vi "HEWH Channel Tester.vi"() -> ()   [LabVIEW 2019]
uses:
  Type Definitions/HEWH Sensor.ctl
  <vilib>/Analysis/NI_AALBase.lvlib
  <vilib>/Utility/file.llb/Write To Spreadsheet File (string).vi
  <vilib>/Utility/file.llb/Write To Spreadsheet File (DBL).vi
  Type Definitions/HEWH Equipment References.ctl
  Type Definitions/HEWH Tank Indicator.ctl
panel:
  out "Use Agilent?":bool
  out "Output Data":string[][](array[string])
  out "Calibration File Array":dbl[][](array[numeric])
  in  "Tab Control 2":T1(tab)
  in  "Panel 1":T2[][](array[typedef])=[[{"Mean"=0.0, " Std"=0.0, "Color Box"=8585007}, {"Mean"=0.0, " Std"=0.0, "Color Box"=8585007}, {"Mean"=0.0, " Std"=0.0, "Color Box"=8585007}, {"Mean"=0.0, " Std"=0.0, "Color Box"=8585007}, {"Mean"=0.0, " Std"=0.0, "Color Box"=8585007}, {"Mean"=0.0, " Std"=0.0, "Color Box"=8585007}], [{"Mean"=0.0, " Std"=0.0, "Color Box"=8585007}, {"Mean"=0.0, " Std"=0.0, "Color Box"=8585007}, {"Mean"=0.0, " Std"=0.0, "Color Box"=8585007}, {"Mean"=0.0, " Std"=0.0, "Color Box"=8585007}, {"Mean"=0.0, " Std"=0.0, "Color Box"=8585007}, {"Mean"=0.0, " Std"=0.0, "Color Box"=8585007}], [{"Mean"=0.0, " Std"=0.0, "Color Box"=8585007}, {"Mean"=0.0, " Std"=0.0, "Color Box"=8585007}, {"Mean"=0.0, " Std"=0.0, "Color Box"=8585007}, {"Mean"=0.0, " Std"=0.0, "Color Box"=8585007}, {"Mean"=0.0, " Std"=0.0, "Color Box"=8585007}, {"Mean"=0.0, " Std"=0.0, "Color Box"=8585007}]]
  in  "Panel 2":T2[][](array[typedef])=[[{"Mean"=0.0, " Std"=0.0, "Color Box"=8585007}, {"Mean"=0.0, " Std"=0.0, "Color Box"=8585007}, {"Mean"=0.0, " Std"=0.0, "Color Box"=8585007}, {"Mean"=0.0, " Std"=0.0, "Color Box"=8585007}, {"Mean"=0.0, " Std"=0.0, "Color Box"=8585007}, {"Mean"=0.0, " Std"=0.0, "Color Box"=8585007}], [{"Mean"=0.0, " Std"=0.0, "Color Box"=8585007}, {"Mean"=0.0, " Std"=0.0, "Color Box"=8585007}, {"Mean"=0.0, " Std"=0.0, "Color Box"=8585007}, {"Mean"=0.0, " Std"=0.0, "Color Box"=8585007}, {"Mean"=0.0, " Std"=0.0, "Color Box"=8585007}, {"Mean"=0.0, " Std"=0.0, "Color Box"=8585007}], [{"Mean"=0.0, " Std"=0.0, "Color Box"=8585007}, {"Mean"=0.0, " Std"=0.0, "Color Box"=8585007}, {"Mean"=0.0, " Std"=0.0, "Color Box"=8585007}, {"Mean"=0.0, " Std"=0.0, "Color Box"=8585007}, {"Mean"=0.0, " Std"=0.0, "Color Box"=8585007}, {"Mean"=0.0, " Std"=0.0, "Color Box"=8585007}]]
  in  "Panel 3":T2[][](array[typedef])=[[{"Mean"=0.0, " Std"=0.0, "Color Box"=8585007}, {"Mean"=0.0, " Std"=0.0, "Color Box"=8585007}, {"Mean"=0.0, " Std"=0.0, "Color Box"=8585007}, {"Mean"=0.0, " Std"=0.0, "Color Box"=8585007}, {"Mean"=0.0, " Std"=0.0, "Color Box"=8585007}, {"Mean"=0.0, " Std"=0.0, "Color Box"=8585007}], [{"Mean"=0.0, " Std"=0.0, "Color Box"=8585007}, {"Mean"=0.0, " Std"=0.0, "Color Box"=8585007}, {"Mean"=0.0, " Std"=0.0, "Color Box"=8585007}, {"Mean"=0.0, " Std"=0.0, "Color Box"=8585007}, {"Mean"=0.0, " Std"=0.0, "Color Box"=8585007}, {"Mean"=0.0, " Std"=0.0, "Color Box"=8585007}], [{"Mean"=0.0, " Std"=0.0, "Color Box"=8585007}, {"Mean"=0.0, " Std"=0.0, "Color Box"=8585007}, {"Mean"=0.0, " Std"=0.0, "Color Box"=8585007}, {"Mean"=0.0, " Std"=0.0, "Color Box"=8585007}, {"Mean"=0.0, " Std"=0.0, "Color Box"=8585007}, {"Mean"=0.0, " Std"=0.0, "Color Box"=8585007}]]
  in  "Num Samples":i32=5
  out "Data Sample":i32
  out "Power":T2={"Mean"=0.0, " Std"=0.0, "Color Box"=8585007}
  out "Tc Down":T2={"Mean"=0.0, " Std"=0.0, "Color Box"=8585007}
  out "Temperatures":T2[](array[typedef])=[{"Mean"=0.0, " Std"=0.0, "Color Box"=8585007}, {"Mean"=0.0, " Std"=0.0, "Color Box"=8585007}, {"Mean"=0.0, " Std"=0.0, "Color Box"=8585007}]
  out "Pressures":T2[](array[typedef])=[{"Mean"=0.0, " Std"=0.0, "Color Box"=8585007}, {"Mean"=0.0, " Std"=0.0, "Color Box"=8585007}, {"Mean"=0.0, " Std"=0.0, "Color Box"=8585007}]
  in  "Time Between Samples (Seconds)":u32
  in  "Tab Control":enum32{"DAQ Test", "Equipment"}(tab)
  in  "Test DAQ":bool
  in  "TC Max OK Val":dbl=400.0
  in  "PSI Min OK":dbl=100.0
  in  "TC Min OK Val":dbl=20.0
  in  "StDev Thresh":dbl=0.2
  in  "PSI Max OK":dbl=400.0
  in  "RTD Max OK":dbl=180.0
  in  "RTD Min OK":dbl=30.0
  in  "Calibration Path":path=path "C:/work/CalibrationFile.csv"
  in  "Equipment":T3={"MW100"="MW100", "AG34970"="A-34972A", "WT210"="WT210"}
  in  "OK":bool
  out "Calibration File?":bool
  in  "Calibration":T4(tab)
  in  "Select Panel to Calibrate":enum16{"Panel 1", "Panel 2", "Panel 3"}(ring)
  in  "Erase Cal File":bool
  in  "Calibrate":bool
  out "Temperature":dbl
  in  "Degrees F":dbl format="%^.3e"
  in  "Test Instrument":bool
  out "Calibration File Path":path
  out "Raw Data":dbl[][](array[numeric]) format="%_6g"
  out "Local Tank Display":T5 {"TC6" format="%.2g"; "TIN" format="%.2g"; "TOUT" format="%.2g"; "TC5" format="%.2g"; "TC4" format="%.2g"; "TC3" format="%.2g"; "TC2" format="%.2g"; "TC1" format="%.2g"}
  in  "error in (no error)":errorcluster
  # "This software is depricated"
  # "HEWH Pannel Channel Tester"
  # "DO NOT MODIFY WITHOUT PROPER PERMISSIONS"
  # "Instructions:\n1. Connect Fluke 525A or 525B (or equivalent) to the selected TC Panel\n2. Connect Fluke GPIB port to computer\n3. Erase old calibration file\n4. Select number of samples (300 default)\n4. Select the appropriate panel\n5. Set the instrument temperature (0,32,90 Degrees F)\n6. Press Calibrate TC's\n7. Repeat step 4 through 6"
  # "Step 1:"
  # "Step 2:"
  # "Step 3:"
  # "Step 5:"
  # "Step 6:"
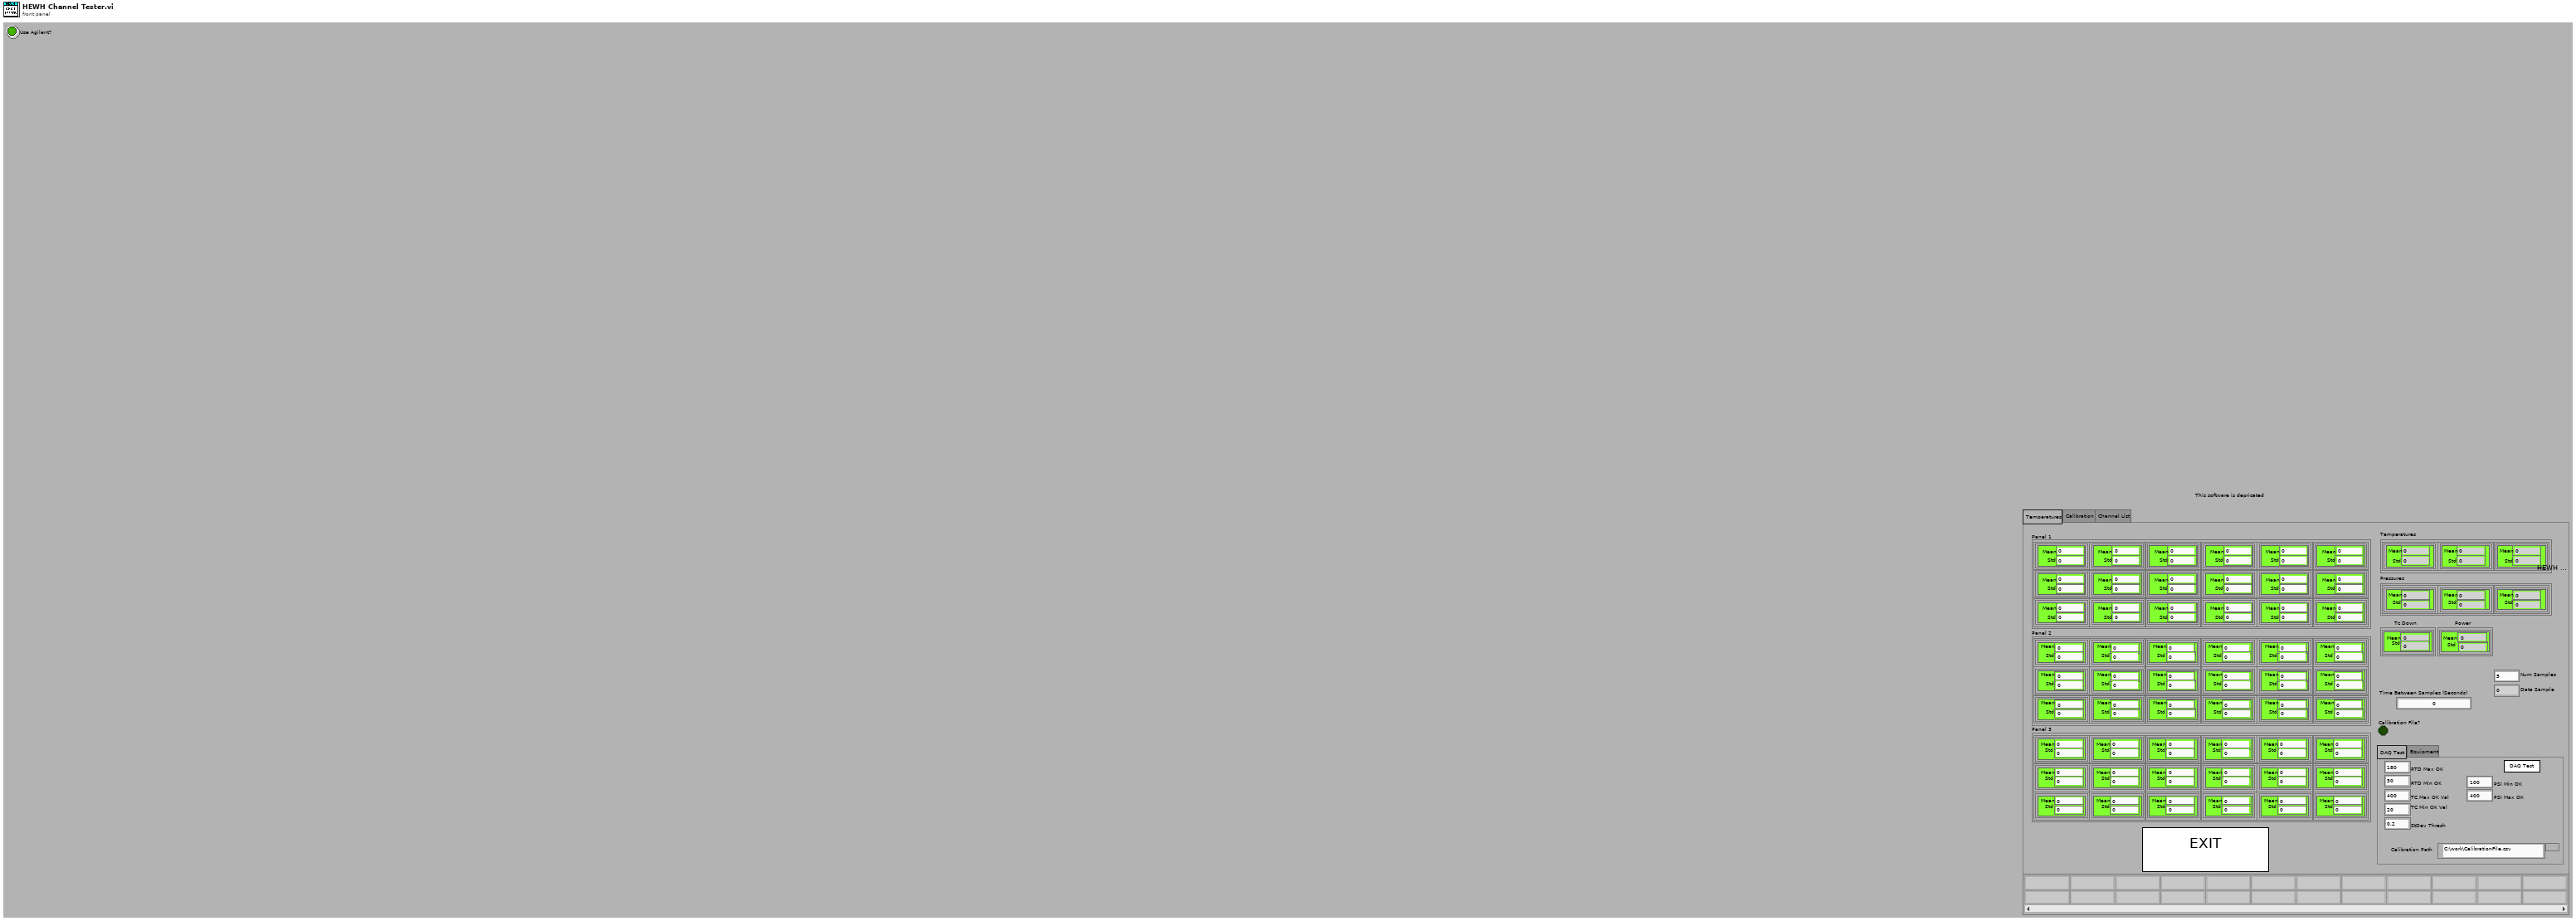
[diagram p1: front panel]
types:
  T1 = enum32{"Temperatures", "Calibration", "Channel List"}
  T2 = typedef "HEWH Sensor.ctl" = cluster{"Mean":dbl, " Std":dbl, "Color Box":u32}
  T3 = typedef "HEWH Equipment References.ctl" = cluster{"MW100":refnum<visa-resource-name>, "AG34970":refnum<visa-resource-name>, "WT210":refnum<visa-resource-name>}
  T4 = enum32{"Calibration Sequence", "Write File", "Debug"}
  T5 = typedef "HEWH Tank Indicator.ctl" = cluster{"TC1":dbl, "TC2":dbl, "TC3":dbl, "TC4":dbl, "TC5":dbl, "TIN":dbl, "TOUT":dbl, "TC6":dbl, "TC6-Color":u32, "TC5-Color":u32, "TC4-Color":u32, "TC3-Color":u32, "TC2-Color":u32, "TC1-Color":u32, "RTD-Out":u32, "RTD-In":u32}
  T6 = enum32{"invalid app kind", "Development System", "Run Time System", "Student Edition", "Embedded LabVIEW", "Evaluation", "Custom"}
  T7 = enum32{"Invalid", "Standard", "Closed", "Hidden", "Minimized", "Maximized"}
  T8 = cluster{"Core":cluster{"Current VI Reference":refnum<vi>, "Close Panel on Exit?":bool}, "Num Samples":i32, "HEWH Power":bool, "Test Data Array":T2[], "Channel List":string}
  T9 = cluster{"Current VI Reference":refnum<vi>, "Close Panel on Exit?":bool}
  T10 = typedef "HEWH Agilent Cluster.ctl" = cluster{"Label":string, "Agilent Channel":string, "Panel ID":string, "Source":string, "Temperature":dbl}
  T11 = typedef "FileVersionInformation.ctl" = cluster{"FileVersion":string, "ProductName":string, "InternalName":string, "CompanyName":string, "LegalCopyright":string, "FileDescription":string}
  T12 = typedef "HEWH Output Information.ctl" = cluster{"TR Number:":string, "Lab ID:":string, "Calibration Array":string[][], "Test Number:":string, "Model:":string, "Serial Number:":string, "Build:":string, "Ambient Temp SetPoint:":string, "Test Station:":string, "Frequency:":string, "Ambient RH:":string, "Comments:":string, "Technician:":string, "Engineer:":string, "Date:":string, "Version:":string, "Computer:":string, "Filename":string, "Heating Mode":string, "FileVersionInfo":T11, "File Initialization Array":string[][], "File Path":path, "Computer IP Address:":string, "Agilent Channel List":string, "Agilent Cluster Array":T13[], "Calibration Coefficients":dbl[][], "Agilent Raw Cluster Array":T13[], "Data Table":string[][], "RLT Station?":bool, "Scan Rate Adjust":dbl, "Start Gallons":dbl, "Last GPM Reading":dbl, "PowerData":T14, "Draw Count":i32, "Draw Patten Setup":T15, "Draw Until Condition":T17, "TC Tree":dbl[], "Starting Temp Decline Temp":dbl, "Full Data Table":string[][], "Max RTD Temp\nDuring Draw":dbl, "Min RTD Temp\nDuring Draw":dbl, "RTD Max Min Array":dbl[][], "Draw Start Time":dbl, "Draw Statistics":dbl[][], "Last Temp Reading":dbl, "Custom Test Array":T18[], "Delay Start Time":dbl, "Condition Cluster Output":T20, "Valve % Open":dbl, "PreDraw Data Table":string[][]}
  T13 = typedef "Agilent Cluster.ctl" = cluster{"Label":string, "Agilent Channel":string, "Panel ID":string, "Source":string, "Temperature":dbl}
  T14 = typedef "PowerData.ctl" = cluster{"Voltage (Volts)":dbl, "Current (Amps)":dbl, "Power (Watts)":dbl, "WattHours (Wh)":dbl, "TC Tree (AVG)":dbl, "Flow Rate (GPM)":dbl, "Gallons (Gal)":dbl, "RTD Out (Deg F)":dbl, "TC Down":dbl}
  T15 = typedef "Draw Pattern Setup.ctl" = cluster{"Dispense Times":dbl[], "Total Gallons Schedule":dbl[], "Flow Rate Schedule ":dbl[], "Incoming Water Temperature":dbl[], "PreDraw Pattern":dbl[][], "Repeat":bool, "24 Hour PreDraw":T16, "Draw Until?":bool[]}
  T16 = typedef "PreDraw.ctl" = enum16{"Zero Pre-Draws", "One Pre- Draws", "Two Pre-Draws", "Three Pre-Draws", ""}
  T17 = typedef "PowerElements.ctl" = cluster{"UE":bool, "LE":bool, "COMP":bool, "FANS":bool}
  T18 = typedef "Custom Test.ctl" = cluster{"Custom Test Value":dbl, "Flow Rate (GPM)":dbl, "Incoming Water  Temperature ":dbl, "Action Type":T19}
  T19 = typedef "Custom Test - Conditions.ctl" = enum16{"", "Set Set Point", "Set to Heat Pump", "Set to Hybrid", "Set to High Demand", "Set to Electric", "Set to Vacation", "Set to Northern Climate", "Check Mode", "Start Test Timer", "Test Timer < Value", "Test Timer > Value", "Check - Test Timer", "Check - Cutout", "Check - Comp ON", "Check - Comp OFF", "Check - Comp & Fan ON", "Check - Comp & Fan OFF", "Check - LE ON", "Check - LE OFF", "Check - UE ON", "Check - UE OFF", "Check - Elapsed Time (sec)", "Check - Mean Tank Temp", "Check - RTD Out Temp Reduction", "Check - RTD Out Temp", "Draw - Elapsed Time (sec)", "Draw - Gallon Target", "Draw - Until Comp", "Draw - Until Comp & Fan", "Draw - Until LE", "Draw - Until UE", "Draw - Any Heat Source", "Draw - Until RTD Out Temp", "Draw - Until RTD Out Temp Reduction", "Draw - Until Mean Tank Temp", "Wait - Cutout", "Wait - Comp ON", "Wait - Comp & Fan ON", "Wait - Comp OFF", "Wait - Comp & Fan OFF", "Wait - LE ON", "Wait - LE OFF", "Wait - UE ON", "Wait - UE OFF", "Wait - Elapsed Time (sec)", "Wait - RTD Out Temp", "Wait - RTD Out Temp Reduction", "Wait - Mean Tank Temp", "Terminate - Comp ON", "Terminate - Comp & Fan ON", "Terminate - Comp OFF", "Terminate - Comp & Fan OFF", "Terminate - LE ON", "Terminate - LE OFF", "Terminate - UE ON", "Terminate - UE OFF", "Terminate - RTD Out Temp", "Terminate - Mean Tank Temp", "Terminate - UE or LE ON", "Terminate - UE or LE OFF", "Terminate - Cutout", "Repeat"}
  T20 = typedef "Termination Condition Cluster.ctl" = cluster{"Decrease RTD Output\nTemperature Bool":bool, "RTD Out Temperature Bool":bool, "Use Time Bool":bool, "RTD Out Temperature":T21, "Decrease Outlet Temperature By (RTD Out)":T21, "Time (Seconds)":T21, "Draw Until Condition":T17, "Start Draw Until Specific Bool":bool, "Return Output Bool":bool, "Draw Until Any Heat Bool":bool, "Mean Tank Temperature Bool":bool, "Mean Tank Temperature":T21, "Comp OFF":bool, "Comp & Fan OFF":bool, "UE OFF":bool, "LE OFF":bool}
  T21 = typedef "DBL.ctl" = dbl
  T22 = typedef "EquipReferences.ctl" = cluster{"MW100":refnum<visa-resource-name>, "AG34970":refnum<visa-resource-name>, "WT210":refnum<visa-resource-name>}
  T23 = typedef "User Controls.ctl" = cluster{"Main Power Control":bool, "Out VLV":enum8{"CLOSE", "OPEN"}, "Expansion Tank?":bool, "In VLV":enum8{"OPEN", "CLOSE"}, "Drain VLV":enum8{"OPEN", "CLOSE"}, "Flow Totalizer Control":bool, "Intellifaucet Temperature":dbl, "Percent Flow":dbl, "Safe Mode":bool, "In VLV B":enum8{"OPEN", "CLOSE"}, "Drain VLV B":enum8{"OPEN", "CLOSE"}, "Out VLV B":enum8{"CLOSE", "OPEN"}, "In VLV C":enum8{"OPEN", "CLOSE"}, "Drain VLV C":enum8{"OPEN", "CLOSE"}, "Out VLV C":enum8{"CLOSE", "OPEN"}, "In VLV D":enum8{"OPEN", "CLOSE"}, "Drain VLV D":enum8{"OPEN", "CLOSE"}, "Out VLV D":enum8{"CLOSE", "OPEN"}, "GEA2?":bool, "Use Agilent?":bool, "Valve Set A":enum16{"Heating", "Purge", "Resting", "Draw"}, "Valve Set B":enum16{"Heating", "Purge", "Resting", "Draw"}, "Valve Set C":enum16{"Heating", "Purge", "Resting", "Draw"}, "Valve Set D":enum16{"Heating", "Purge", "Resting", "Draw"}}
  T24 = typedef "PowerAnalyzer.ctl" = enum16{"OSI", "WT210"}
  T25 = cluster{"Core":cluster{"Current VI Reference":refnum<vi>, "Close Panel on Exit?":bool}, "FileVersionInfo Out 2":T11, "Data File Directory":path, "FileInit Cluster":T12, "Equipment VISA":T22, "User Controls":T23, "POWER":T17, "Save Data":string[][], "Calibration File":path, "Power Analyzer":T24}
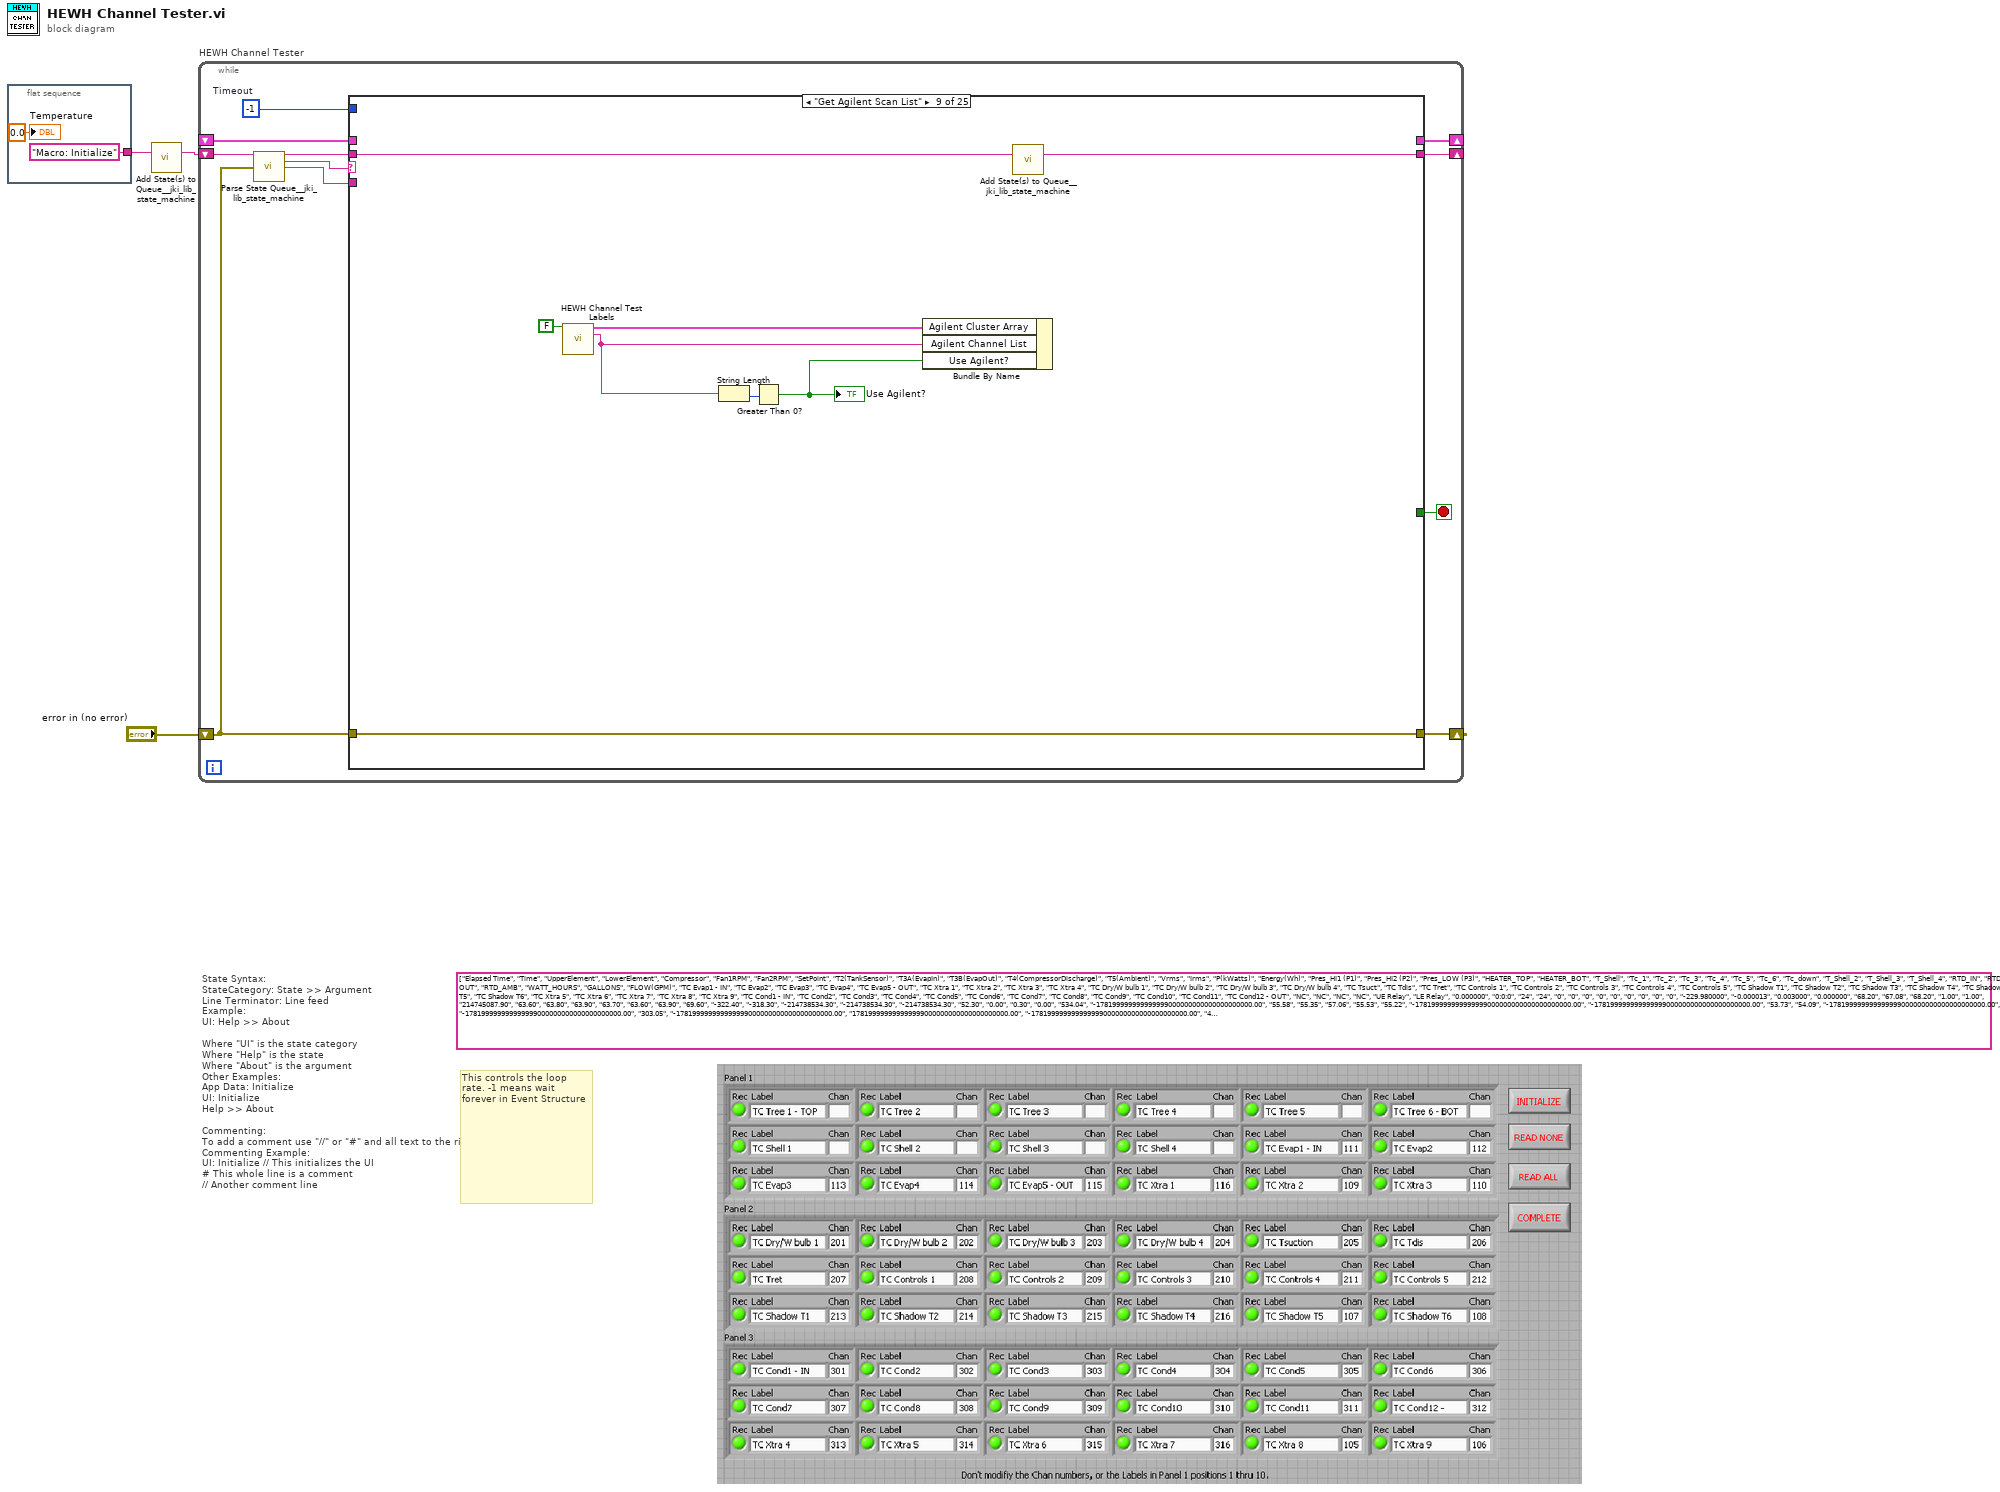
[diagram p0: block diagram]
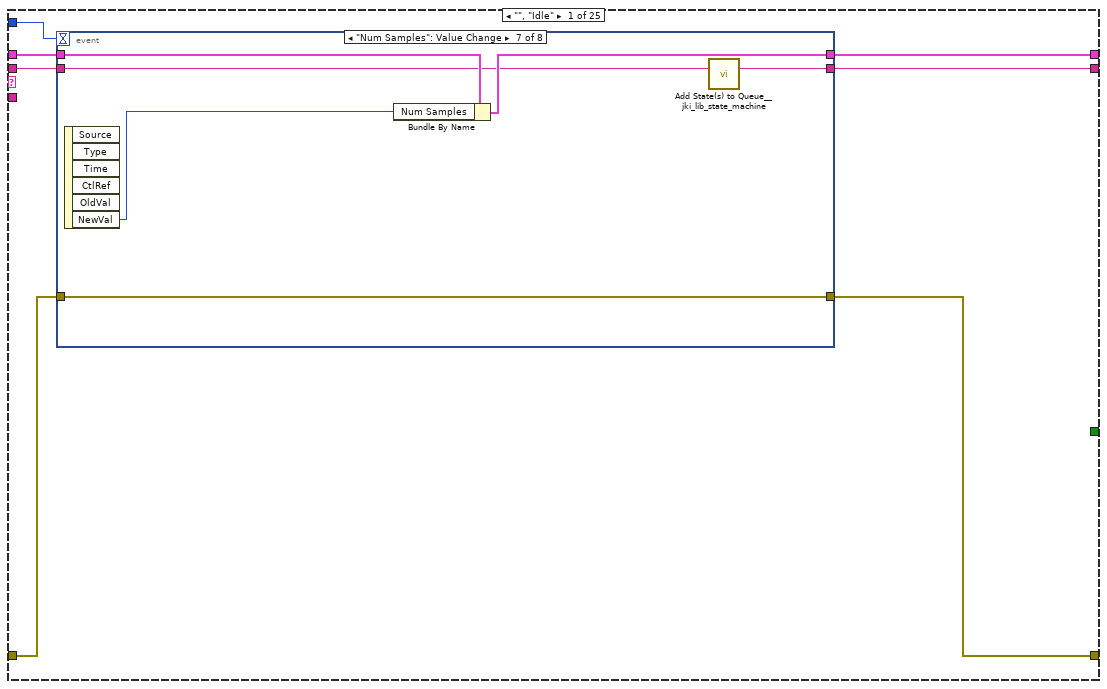
[diagram p2: hidden frame]
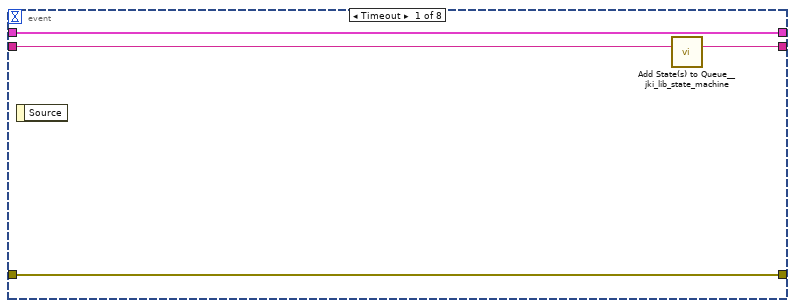
[diagram p3: hidden frame]
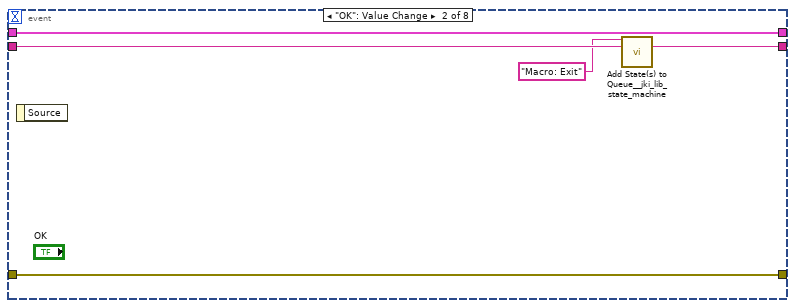
[diagram p4: hidden frame]
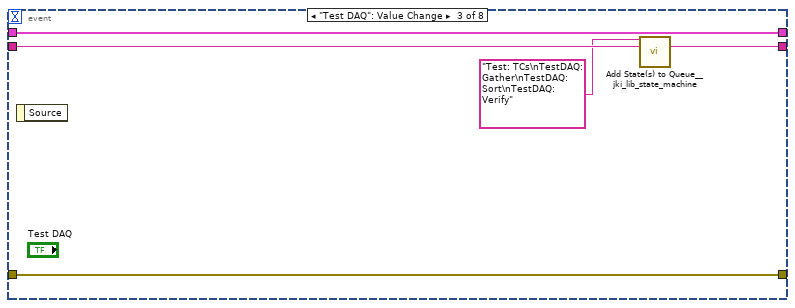
[diagram p5: hidden frame]
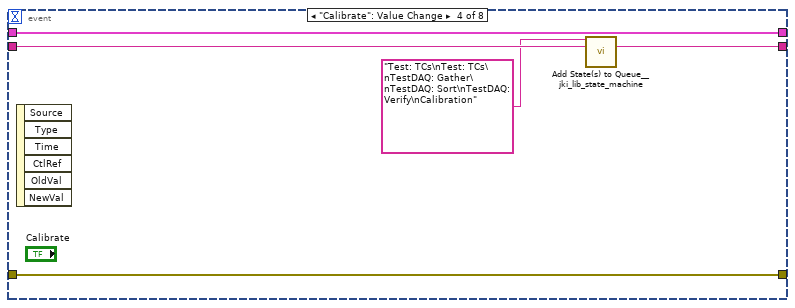
[diagram p6: hidden frame]
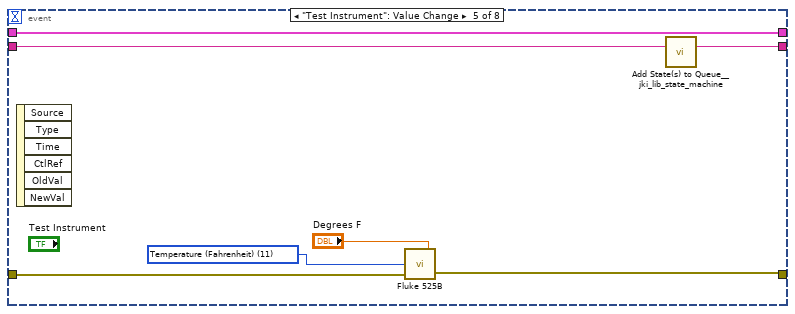
[diagram p7: hidden frame]
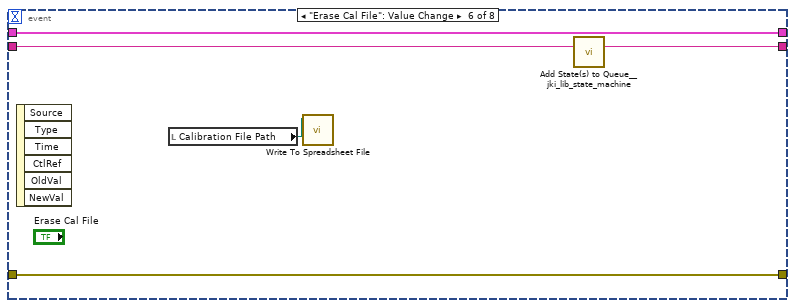
[diagram p8: hidden frame]
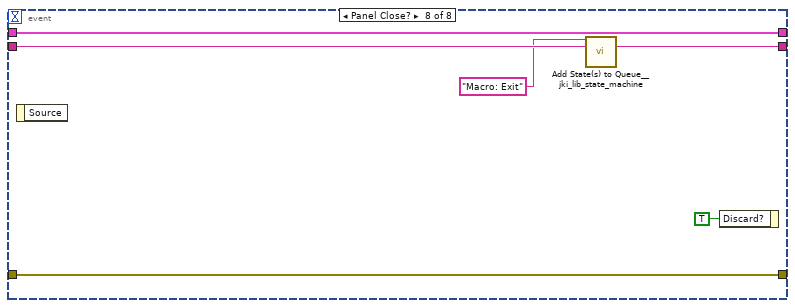
[diagram p9: hidden frame]
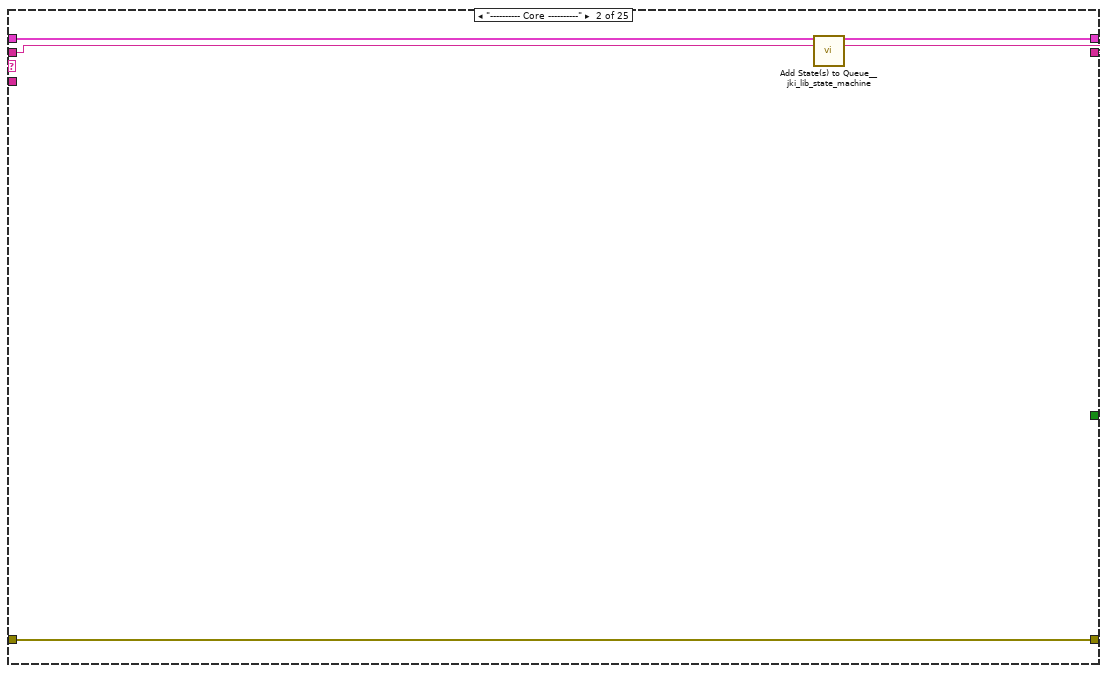
[diagram p10: hidden frame]
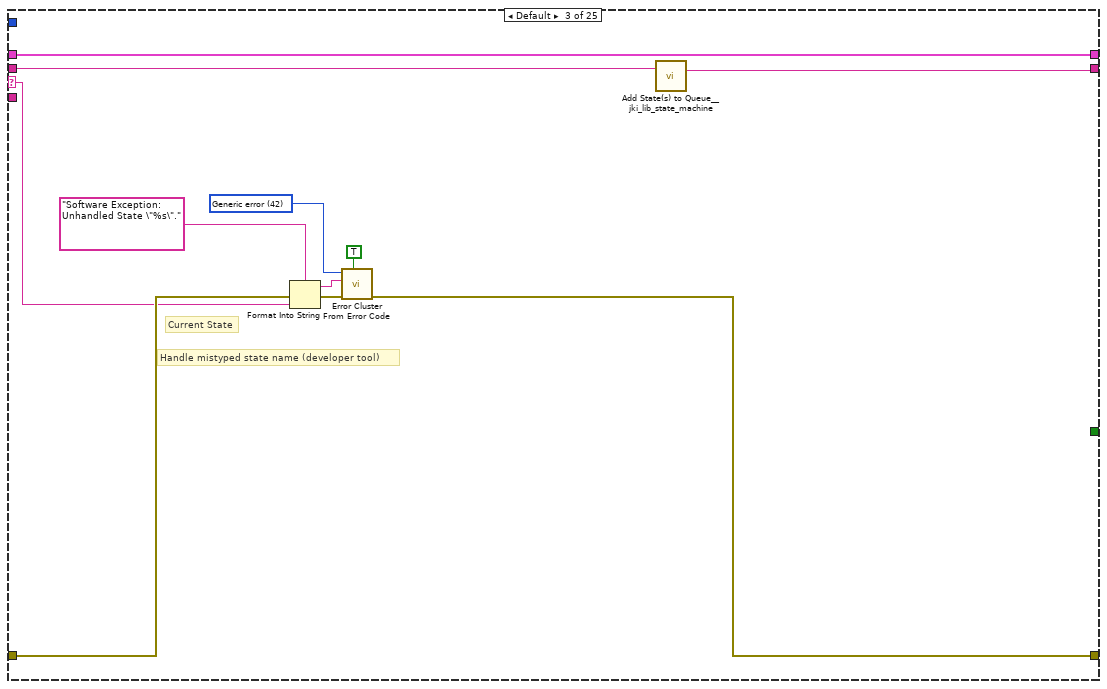
[diagram p11: hidden frame]
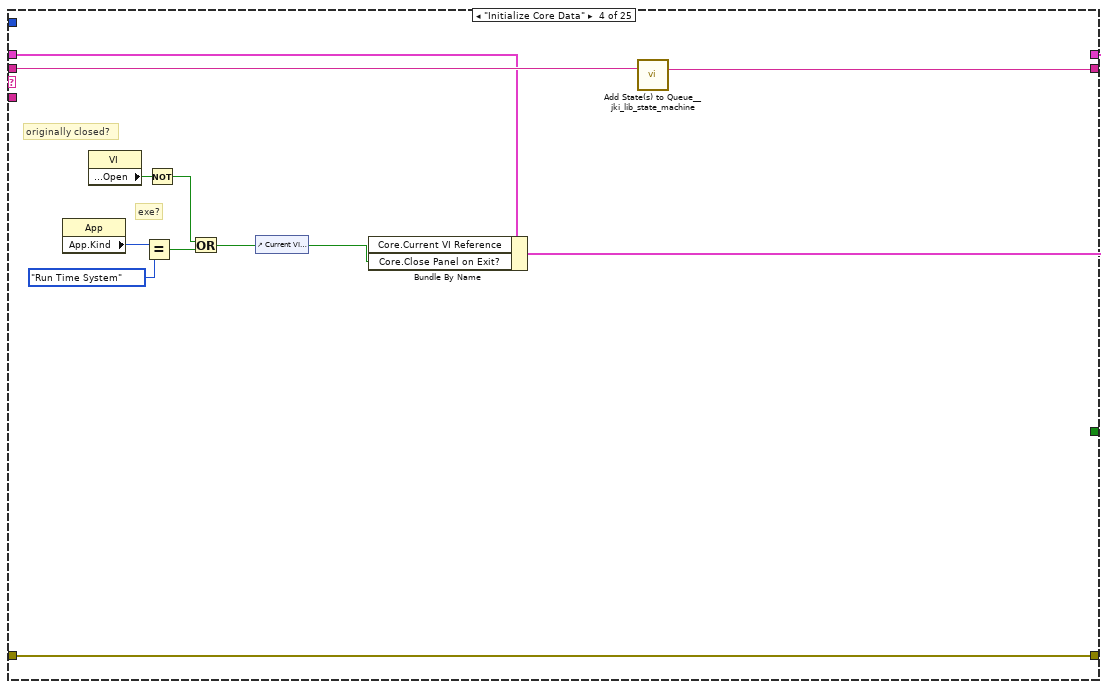
[diagram p12: hidden frame]
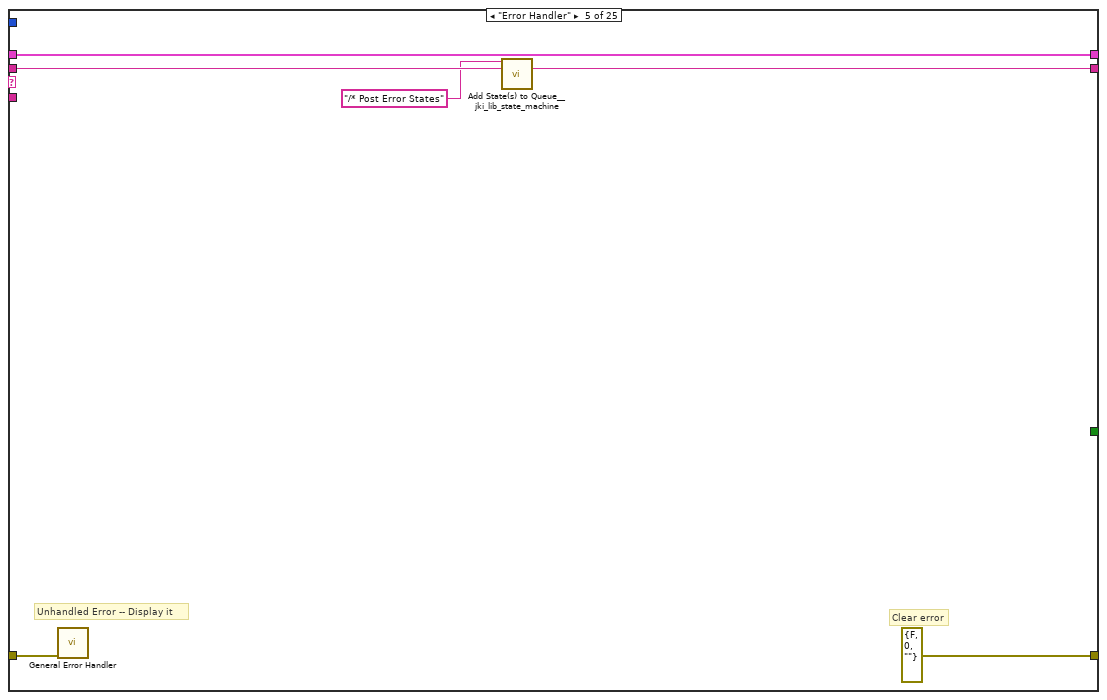
[diagram p13: hidden frame]
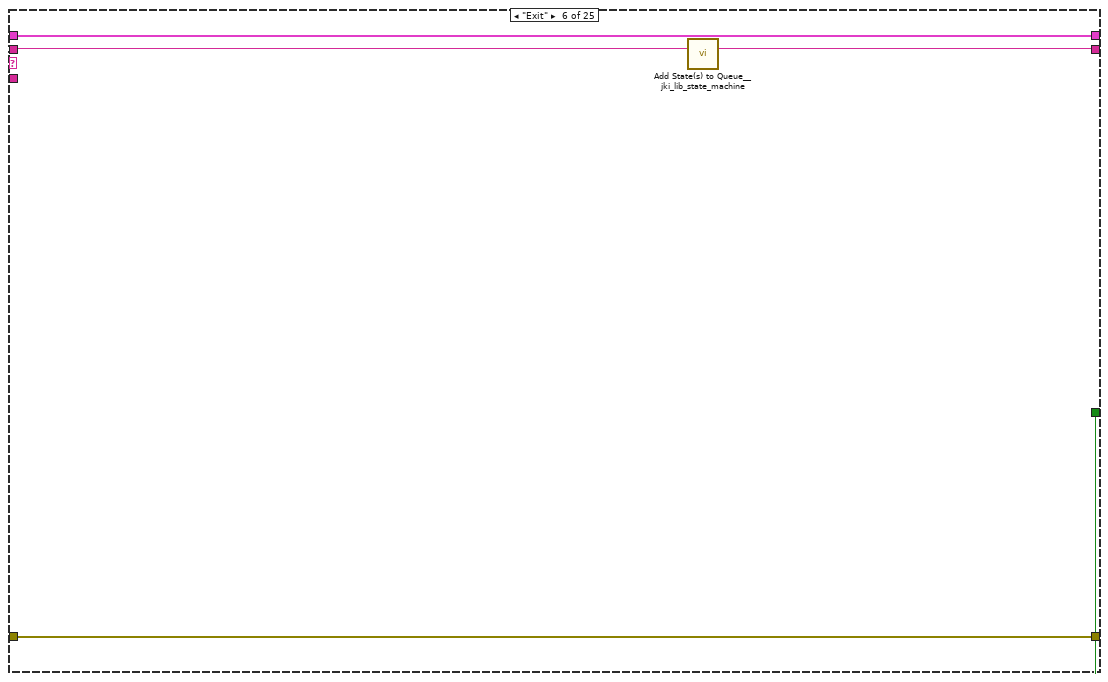
[diagram p14: hidden frame]
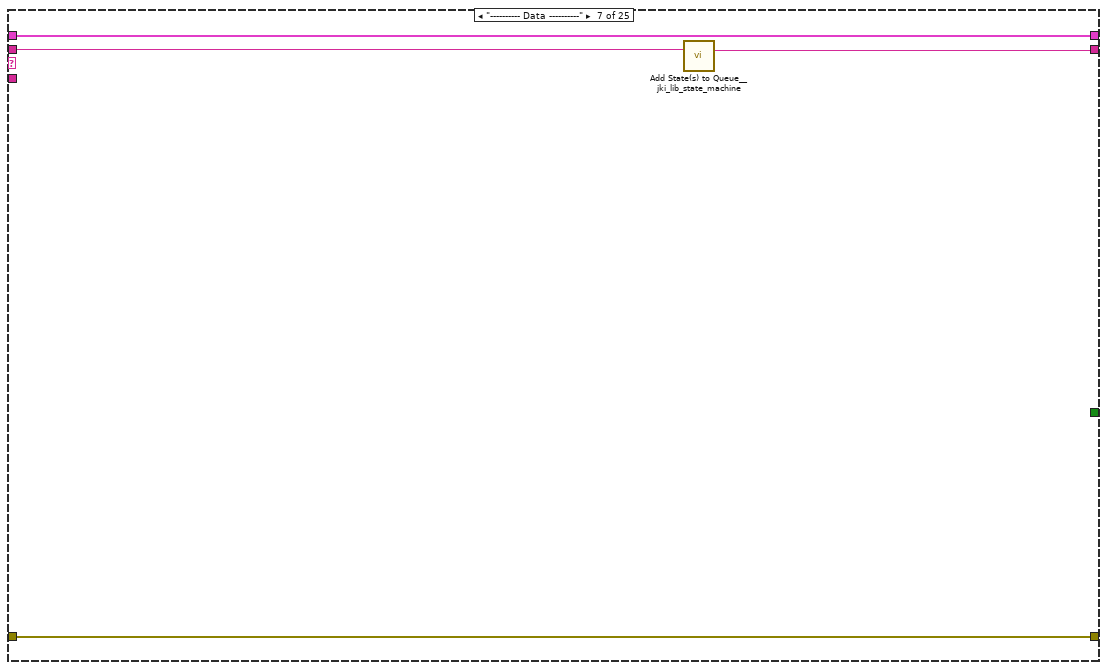
[diagram p15: hidden frame]
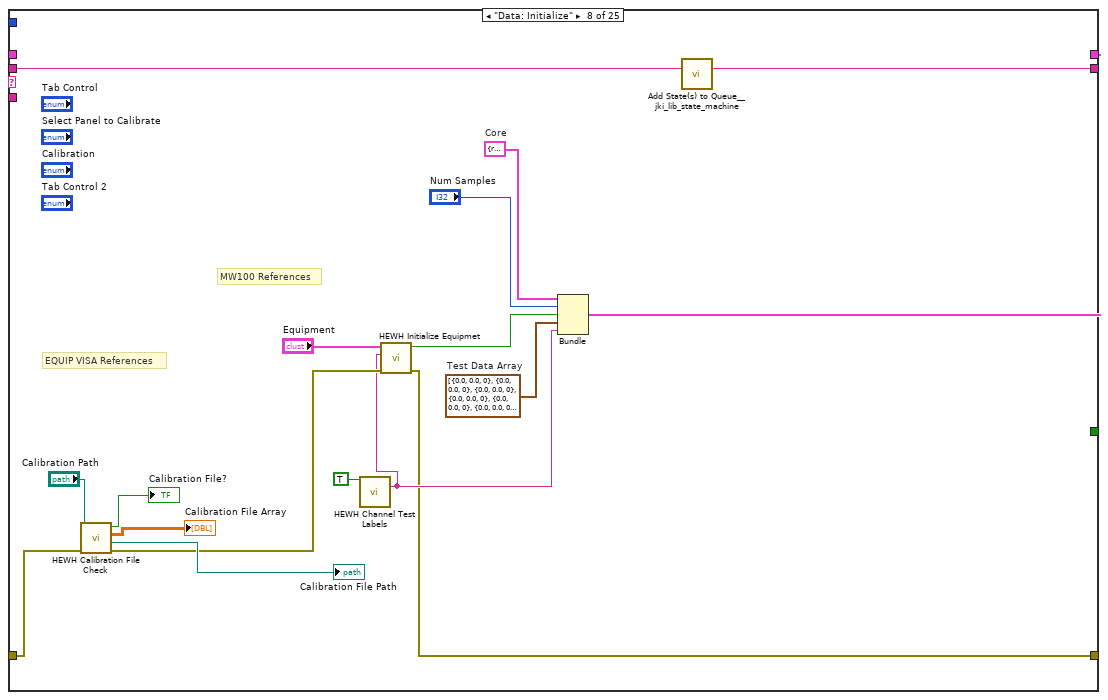
[diagram p16: hidden frame]
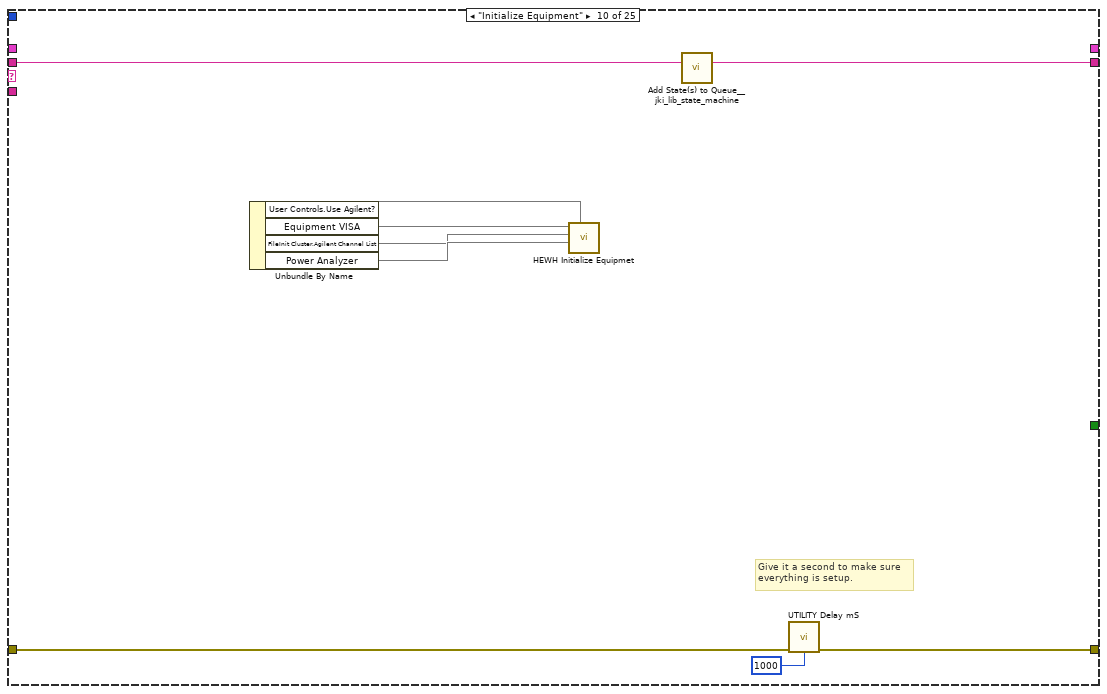
[diagram p17: hidden frame]
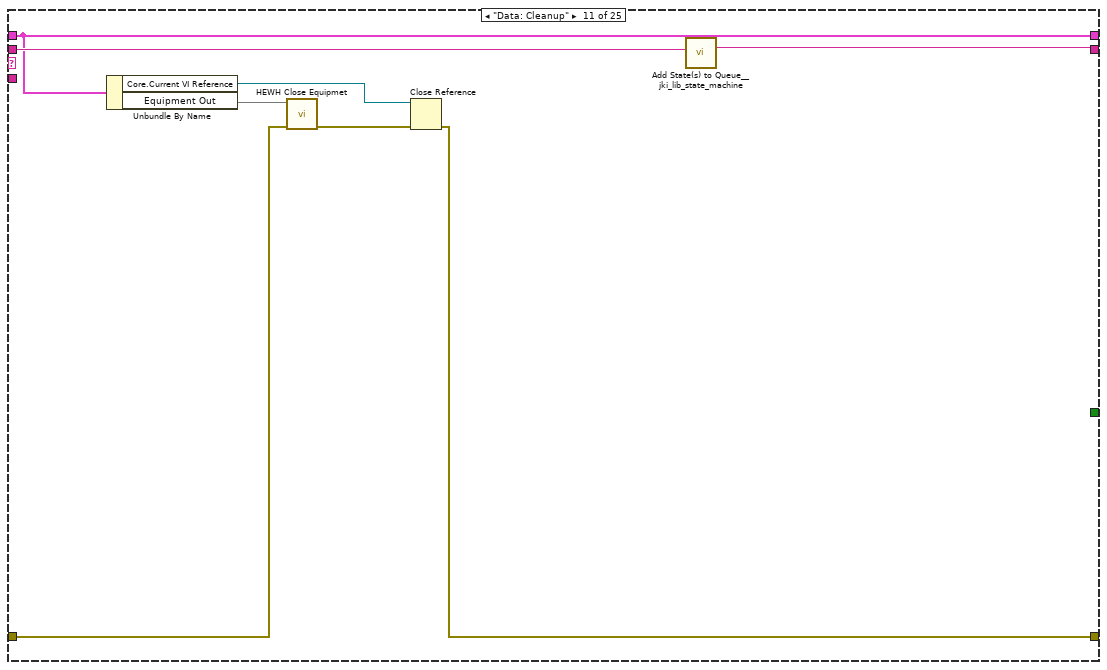
[diagram p18: hidden frame]
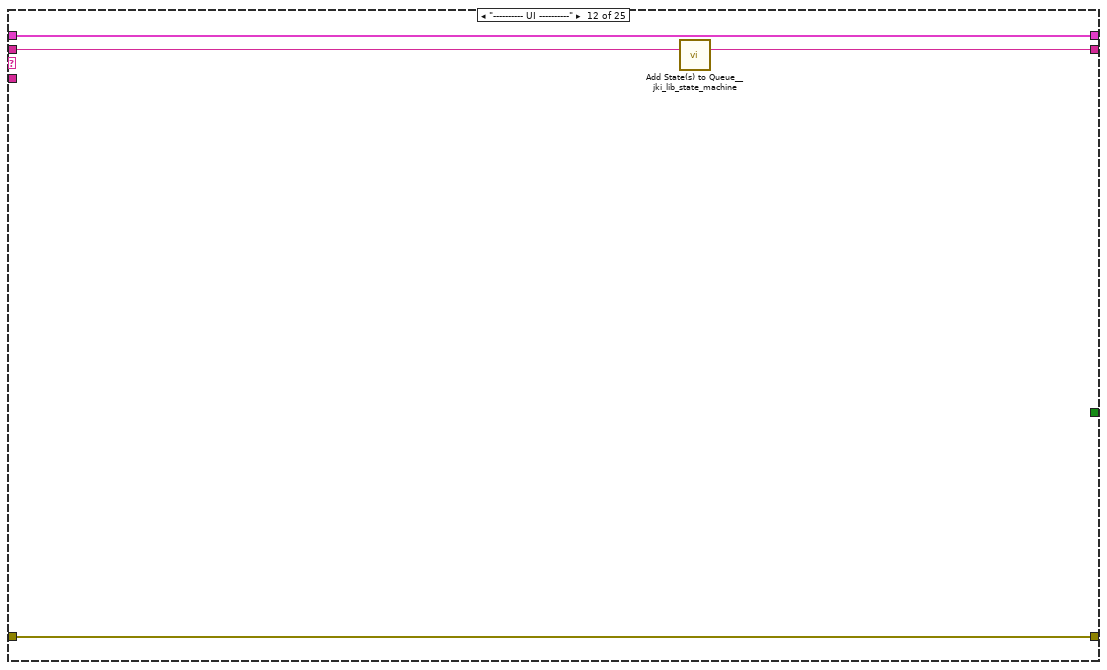
[diagram p19: hidden frame]
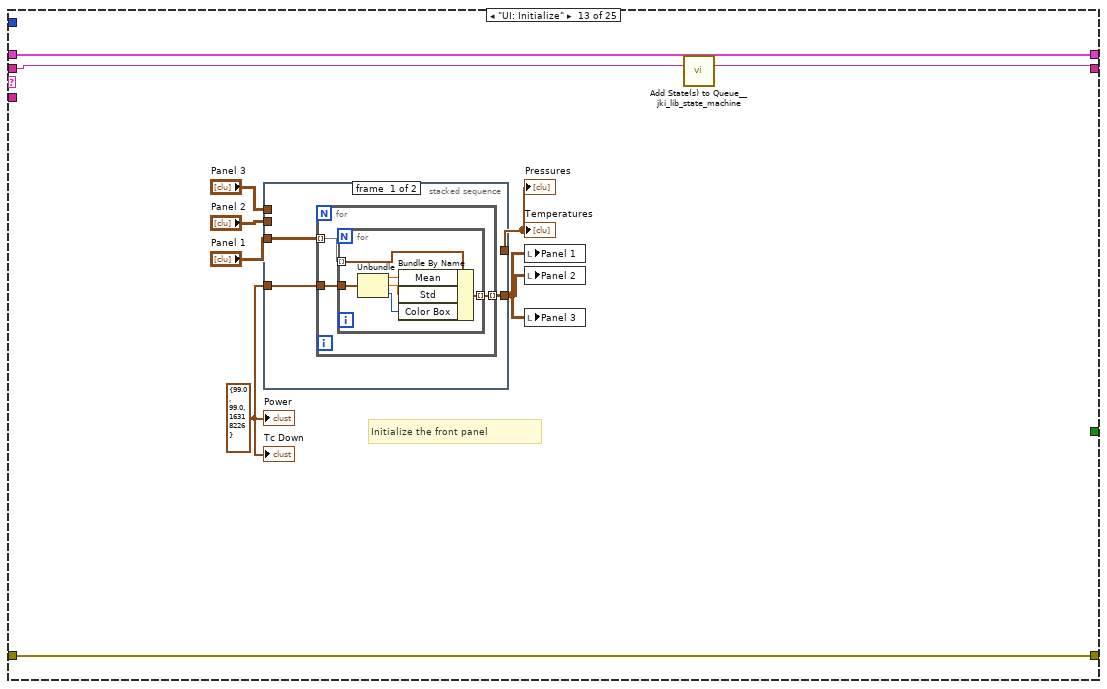
[diagram p20: hidden frame]
diagram:
  (unwired) string[][] [["Elapsed Time", "Time", "UpperElement", "LowerElement", "Compressor", "Fan1RPM", "Fan2RPM", "SetPoint", "T2(TankSensor)", "T3A(EvapIn)", "T3B(EvapOut)", "T4(CompressorDischarge)", "T5(Ambient)", "Vrms", "Irms", "P(kWatts)", "Energy(Wh)", "Pres_HI1 (P1)", "Pres_HI2 (P2)", "Pres_LOW (P3)", "HEATER_TOP", "HEATER_BOT", "T_Shell", "Tc_1", "Tc_2", "Tc_3", "Tc_4", "Tc_5", "Tc_6", "Tc_down", "T_Shell_2", "T_Shell_3", "T_Shell_4", "RTD_IN", "RTD_OUT", "RTD_AMB", "WATT_HOURS", "GALLONS", "FLOW(GPM)", "TC Evap1 - IN", "TC Evap2", "TC Evap3", "TC Evap4", "TC Evap5 - OUT", "TC Xtra 1", "TC Xtra 2", "TC Xtra 3", "TC Xtra 4", "TC Dry/W bulb 1", "TC Dry/W bulb 2", "TC Dry/W bulb 3", "TC Dry/W bulb 4", "TC Tsuct", "TC Tdis", "TC Tret", "TC Controls 1", "TC Controls 2", "TC Controls 3", "TC Controls 4", "TC Controls 5", "TC Shadow T1", "TC Shadow T2", "TC Shadow T3", "TC Shadow T4", "TC Shadow T5", "TC Shadow T6", "TC Xtra 5", "TC Xtra 6", "TC Xtra 7", "TC Xtra 8", "TC Xtra 9", "TC Cond1 - IN", "TC Cond2", "TC Cond3", "TC Cond4", "TC Cond5", "TC Cond6", "TC Cond7", "TC Cond8", "TC Cond9", "TC Cond10", "TC Cond11", "TC Cond12 - OUT", "NC", "NC", "NC", "NC", "UE Relay", "LE Relay"], ["0.000000", "0:0:0", "24", "24", "0", "0", "0", "0", "0", "0", "0", "0", "0", "-229.980000", "-0.000013", "0.003000", "0.000000", "68.20", "67.08", "68.20", "1.00", "1.00", "214745087.90", "63.60", "63.80", "63.90", "63.70", "63.60", "63.90", "69.60", "-322.40", "-318.30", "-214738534.30", "-214738534.30", "-214738534.30", "52.30", "0.00", "0.30", "0.00", "534.04", "-178199999999999999000000000000000000000.00", "55.58", "55.35", "57.06", "55.53", "55.22", "-178199999999999999000000000000000000000.00", "-178199999999999999000000000000000000000.00", "53.73", "54.09", "-178199999999999999000000000000000000000.00", "-178199999999999999000000000000000000000.00", "303.05", "-178199999999999999000000000000000000000.00", "178199999999999999000000000000000000000.00", "-178199999999999999000000000000000000000.00", "460.73", "626.99", "-178199999999999999000000000000000000000.00", "178199999999999999000000000000000000000.00", "-178199999999999999000000000000000000000.00", "131.37", "178199999999999999000000000000000000000.00", "-178199999999999999000000000000000000000.00", "-178199999999999999000000000000000000000.00", "409.13", "259.86", "-178199999999999999000000000000000000000.00", "178199999999999999000000000000000000000.00", "-178199999999999999000000000000000000000.00", "-57.06", "62.09", "61.89", "61.87", "62.14", "62.63", "178199999999999999000000000000000000000.00", "-178199999999999999000000000000000000000.00", "178199999999999999000000000000000000000.00", "-70.58", "-178199999999999999000000000000000000000.00", "178199999999999999000000000000000000000.00", "-178199999999999999000000000000000000000.00", "393.52", "116.86", "83.34", "59.96", "0", "0"]] ("Output Data")
  # "State Syntax:\nStateCategory: State >> Argument\nLine Terminator: Line feed\nExample:\nUI: Help >> About\n\nWhere \"UI\" is the state category\nWhere \"Help\" is the state\nWhere \"About\" is the argument\nOther Examples:\nApp Data: Initialize\nUI: Initialize\nHelp >> About\n\nCommenting:\nTo add a comment use \"//\" or \"#\" and all text to the right will be ignored\nCommenting Example:\nUI: Initialize // This initializes the UI\n# This whole line is a comment\n// Another comment line"
  # "This controls the loop rate. -1 means wait forever in Event Structure"
  n1 = flat-sequence {
    tunnel: ["Macro: Initialize"] -> w1
    frame #0 {
      "Temperature" <- 0.0 ("Temp Counter")
    }
  }
  n2 = call <vilib>:"Add State(s) to Queue__jki_lib_state_machine.vi"("State(s) in (\"\")"=w1) -> ("States Out"=w3:string)  [unwired: 14 in]
  n3 = while "HEWH Channel Tester" {
    shift-right: [w9] -> _
    shift-left: _ -> [w8]
    shift-right: [w12] -> _
    shift-left: "error in (no error)" -> [w6]
    shift-right: [w11] -> _
    shift-left: w3 -> [w13]
    stop <- w10 stop-if-true
    w7 = -1  # Timeout
    # "Template Copyright © 2008 JKI - http://jkisoft.com/state-machine"
    n4 = call <vilib>:"Parse State Queue__jki_lib_state_machine.vi"("State Queue"=w13, "Error In (no error)"=w6) -> ("Remaining States"=w15:string, "Current State"=w16:string, "Arguments"=w14:string)  [unwired: 11 in]
    n5 = case shown="\"Get Agilent Scan List\"" w16 {
      selector: w16 -> [_ _ w73 _ _ _ _ _ _ _ _ _ _ _ _ _ _ _ _ _ _ _ _ _ _]
      tunnel: w15 -> [w23 w70 w71 w93 w99 w104 w108 w125 w133 w143 w151 w155 w165 w188 w199 w225 w230 w240 w244 w248 w252 w263 w289 w374 w412]
      tunnel: w14 -> [_ _ _ _ _ _ _ _ _ _ _ _ _ w183 w193 _ _ _ _ _ _ _ _ _ _]
      tunnel: w8 -> [w21 w67 w75 w84 w96 w102 w105 _ _ _ w147 w152 w163 w186 w195 w222 w227 w237 w241 w245 w249 w259 w286 w371 w410]
      tunnel: [w20 w68 w77 w90 errorcluster {"status"=FALSE, "code"=0, "source"=""} ("error out") w101 w106 w110 w131 w134 w148 w153 w162 w184 w196 w223 w228 w238 w242 w246 w250 w261 w287 w372 w406] -> w12
      tunnel: w6 -> [w19 w68 w76 w90 w95 w101 w106 w114 w131 w135 w144 w153 w162 w185 w197 w223 w228 w238 w242 w246 w250 w255 w287 w372 w407]
      tunnel: [w22 w69 w72 w92 w98 w103 w107 w124 w132 w142 w150 w154 w164 w187 w198 w224 w229 w239 w243 w247 w251 w262 w288 w373 w411] -> w11
      tunnel: [_ _ _ _ _ TRUE _ _ _ _ _ _ _ _ _ _ _ _ _ _ _ _ _ _ _] -> w10
      tunnel: [w18 w67 w75 w91 w96 w102 w105 w123 _ _ w147 w152 w163 w186 w195 w222 w227 w237 w241 w245 w249 w257 w286 w371 w410] -> w9
      tunnel: w7 -> [w17 _ _ _ _ _ _ _ _ _ _ _ _ _ _ _ _ _ _ _ _ _ _ _ _]
      frame "", "Idle" {
        n6 = event shown="[6] \"Num Samples\": Value Change" {
          selector: _ -> [_ _ _ _ _ _ _ _]
          dyn-events: _ -> [_ _ _ _ _ _ _ _]
          timeout: w17 -> [_ _ _ _ _ _ _ _]
          tunnel: w23 -> [w27 w32 w37 w42 w48 w53 w58 w66]
          tunnel: [w26 w31 w36 w41 w49 w52 w57 w65] -> w22
          tunnel: w21 -> [w24 w29 w34 w39 w47 w54 w60 w63]
          tunnel: [w25 w30 w35 w40 w43 w51 w56 w64] -> w20
          tunnel: w19 -> [w25 w30 w35 w40 w44 w51 w56 w64]
          tunnel: [w24 w29 w34 w39 w47 w54 w59 w63] -> w18
          event Timeout {
            n7 = event-data() -> ()  [unwired: 1 in, 1 out]
            n8 = call <vilib>:"Add State(s) to Queue__jki_lib_state_machine.vi"("State(s) in (\"\")"=w27) -> ("States Out"=w26:string)  [unwired: 14 in]
          }
          event "OK": Value Change {
            n9 = event-data() -> ()  [unwired: 1 in, 1 out]
            n10 = call <vilib>:"Add State(s) to Queue__jki_lib_state_machine.vi"("State(s) in Front (\"\")"="Macro: Exit", "State(s) in (\"\")"=w32) -> ("States Out"=w31:string)  [unwired: 13 in]
          }
          event "Test DAQ": Value Change {
            n11 = event-data() -> ()  [unwired: 1 in, 1 out]
            n12 = call <vilib>:"Add State(s) to Queue__jki_lib_state_machine.vi"("State(s) in Front (\"\")"="Test: TCs\nTestDAQ: Gather\nTestDAQ: Sort\nTestDAQ: Verify", "State(s) in (\"\")"=w37) -> ("States Out"=w36:string)  [unwired: 13 in]
          }
          event "Calibrate": Value Change {
            n13 = event-data() -> ()  [unwired: 1 in, 6 out]
            n14 = call <vilib>:"Add State(s) to Queue__jki_lib_state_machine.vi"("State(s) in Front (\"\")"="Test: TCs\nTest: TCs\nTestDAQ: Gather\nTestDAQ: Sort\nTestDAQ: Verify\nCalibration", "State(s) in (\"\")"=w42) -> ("States Out"=w41:string)  [unwired: 13 in]
          }
          event "Test Instrument": Value Change {
            w45 = u32 11 items=["Amplitude", "Volts dc or update volts ac", "Volts ac dBm update", "Volts ac or volts dc with 0 Hz", "Volts ac in dBm", "Current dc or update current ac", "Current ac", "Update frequency", "Resistance", "Capacitance", "Temperature (Celsius)", "Temperature (Fahrenheit)", "Power dc or update power ac", "Power ac", "Dual volts dc or update dual ac", "Dual volts ac in volts", "Power ac in dBm update", "Power ac in dBm", "Dual volts ac in dBm update", "Dual volts ac in dBm"] ("Output Value(s) (3: Volts ac or volts dc with 0 Hz)")
            n15 = event-data() -> ()  [unwired: 1 in, 6 out]
            n16 = call "Fluke 525B.vi"("Primary Value (1.234)"="Degrees F", "error in (no error)"=w44, "Output Value(s) (3: Volts ac or volts dc with 0 Hz)"=w45) -> ("error out"=w43:errorcluster)  [unwired: 1 in]
            n17 = call <vilib>:"Add State(s) to Queue__jki_lib_state_machine.vi"("State(s) in (\"\")"=w48) -> ("States Out"=w49:string)  [unwired: 14 in]
          }
          event "Erase Cal File": Value Change {
            n18 = event-data() -> ()  [unwired: 1 in, 6 out]
            n19 = local read "Calibration File Path"() -> (w50:path)
            n20 = call-poly <vilib>:"Write To Spreadsheet File.vi"("file path (dialog if empty)"=w50) -> ()  [unwired: 7 in, 1 out]
            n21 = call <vilib>:"Add State(s) to Queue__jki_lib_state_machine.vi"("State(s) in (\"\")"=w53) -> ("States Out"=w52:string)  [unwired: 14 in]
          }
          event "Num Samples": Value Change {
            n22 = event-data() -> ("NewVal"=w55:i32)  [unwired: 1 in, 5 out]
            n23 = Bundle By Name(cluster=w60, "Num Samples"=w55) -> (w59:T8)
            n24 = call <vilib>:"Add State(s) to Queue__jki_lib_state_machine.vi"("State(s) in (\"\")"=w58) -> ("States Out"=w57:string)  [unwired: 14 in]
          }
          event Panel Close? {
            n25 = event-data() -> ()  [unwired: 1 in, 1 out]
            n26 = call <vilib>:"Add State(s) to Queue__jki_lib_state_machine.vi"("State(s) in Front (\"\")"="Macro: Exit", "State(s) in (\"\")"=w66) -> ("States Out"=w65:string)  [unwired: 13 in]
            n27 = event-data("Discard?"=TRUE) -> ()  [unwired: 1 in, 1 out]
          }
        }
      }
      frame "---------- Core ----------" {
        n28 = call <vilib>:"Add State(s) to Queue__jki_lib_state_machine.vi"("State(s) in (\"\")"=w70) -> ("States Out"=w69:string)  [unwired: 14 in]
      }
      frame Default {
        w80 = 42 items=["No error", "Argument error", "Memory is full", "Out of zone", "End of file", "File already open", "Generic file I/O error", "File not found", "File permission error", "Disk is full", "Duplicate path", "Too many files open", "System feature not enabled", "Resource file not found", "Cannot add resource", "Resource not found", "Image not found", "Image memory error", "Pen does not exist", "Config type invalid", "Config token not found", "Config parse error", "Config memory error", "Bad external code format", "Bad external code offset", "External code not present", "Null window", "Destroy window error", "Null menu", "Print aborted", "Bad print record", "Print driver error", "Windows error during printing", "Memory error during printing", "Print dialog error", "Generic print error", "Invalid device refnum", "Device not found", "Device parameter error", "Device unit error", "Cannot open device", "Device call aborted", "Generic error", "Cancelled by user", "Object ID too low", "Object ID too high", "Object not in heap", "Unknown heap", "Unknown object (invalid DefProc)", "Unknown object (DefProc not in table)", "Message out of range", "Invalid (null) method", "Unknown message", "Manager call not supported", "Bad address", "Network operation in progress", "Network operation timed out", "Connection is busy", "Network attribute not supported", "Network error", "Address in use", "System out of memory", "Connection aborted", "Connection refused", "Not connected", "Already connected", "Connection closed", "Initialization error (interapplication manager)", "Bad occurrence", "Wait on unbound occurrence handler", "Occurrence queue overflow", "Datalog type conflict", "Unused", "Unrecognized type (interapplication manager)", "Memory corrupt", "Failed to make temporary DLL", "Old CIN version", "Drag socket not found", "Failed to load drop-object", "Failed to register OLE object", "Failed to release OLE object", "Format specifier type mismatch", "Unknown format specifier", "Too few format specifiers", "Too many format specifiers", "Scan failed", "Newer CIN version", "Error converting to variant", "Runtime menu error", "Password tampered", "Variant attribute not found", "Incompatible variant data type", "Event data is not available", "Event Store is not present", "Occurrence is not found", "Event Queue is not created", "Event info is not available", "Refnum passed is NULL", "Error retrieving Class GUID", "Error retrieving CoClass GUID", "Error retrieving TypeLib GUID.", "Bad built application magic bytes.", "Specific driver is different from the specific driver associated with the Logical Name.", "There is no session opened to the class driver.", "Max Error", "MAX - Error with config objects", "MAX - Error loading configuration", "MAX - Group not supported"]
        # "Current State"
        # "Handle mistyped state name (developer tool)"
        n29 = Format Into String(format string="Software Exception: Unhandled State \"%s\"." ("message"), error in=w76, w73) -> (resulting string=w79:string, error out=w78:errorcluster)  [unwired: 1 in]
        n30 = call <vilib>:"Error Cluster From Error Code.vi"("show call chain? (False)"=TRUE, "error in (no error)"=w78, "error message (\"\")"=w79, "error code (0)"=w80) -> ("error out"=w77:errorcluster)  [unwired: 5 in]
        n31 = call <vilib>:"Add State(s) to Queue__jki_lib_state_machine.vi"("State(s) in (\"\")"=w71) -> ("States Out"=w72:string)  [unwired: 14 in]
      }
      frame "Initialize Core Data" {
        # "originally closed?"
        # "exe?"
        n32 = property class="App"() -> ("App.Kind"=w88:T6)  [unwired: 2 in, 2 out]
        n33 = property class="VI"() -> ("Front Panel.Open"=w89:bool)  [unwired: 2 in, 2 out]
        n34 = Equal?(x=w88, y=T6."Run Time System" ("Application:Kind")) -> (x = y?=w85:bool)
        n35 = Not(x=w89) -> (.not. x?=w86:bool)
        n36 = Or(x=w86, y=w85) -> (x .or. y?=w83:bool)
        n37 = control-ref of="Current VI Reference"() -> (w82:refnum<vi>)
        n38 = Bundle By Name(cluster=w84, "Core.Current VI Reference"=w82, "Core.Close Panel on Exit?"=w83) -> (w91:T8)
        n39 = call <vilib>:"Add State(s) to Queue__jki_lib_state_machine.vi"("State(s) in (\"\")"=w93) -> ("States Out"=w92:string)  [unwired: 14 in]
      }
      frame "Error Handler" {
        # "Unhandled Error -- Display it"
        # "Clear error"
        n40 = call <vilib>:"General Error Handler.vi"("error in (no error)"=w95) -> ()  [unwired: 10 in, 5 out]
        n41 = call <vilib>:"Add State(s) to Queue__jki_lib_state_machine.vi"("State(s) in Front (\"\")"="/* Post Error States", "State(s) in (\"\")"=w99) -> ("States Out"=w98:string)  [unwired: 13 in]
      }
      frame "Exit" {
        n42 = call <vilib>:"Add State(s) to Queue__jki_lib_state_machine.vi"("State(s) in (\"\")"=w104) -> ("States Out"=w103:string)  [unwired: 14 in]
      }
      frame "---------- Data ----------" {
        n43 = call <vilib>:"Add State(s) to Queue__jki_lib_state_machine.vi"("State(s) in (\"\")"=w108) -> ("States Out"=w107:string)  [unwired: 14 in]
      }
      frame "Data: Initialize" {
        w119 = T2[] [{"Mean"=0.0, " Std"=0.0, "Color Box"=0}, {"Mean"=0.0, " Std"=0.0, "Color Box"=0}, {"Mean"=0.0, " Std"=0.0, "Color Box"=0}, {"Mean"=0.0, " Std"=0.0, "Color Box"=0}, {"Mean"=0.0, " Std"=0.0, "Color Box"=0}, {"Mean"=0.0, " Std"=0.0, "Color Box"=0}, {"Mean"=0.0, " Std"=0.0, "Color Box"=0}, {"Mean"=0.0, " Std"=0.0, "Color Box"=0}, {"Mean"=0.0, " Std"=0.0, "Color Box"=0}, {"Mean"=0.0, " Std"=0.0, "Color Box"=0}, {"Mean"=0.0, " Std"=0.0, "Color Box"=0}, {"Mean"=0.0, " Std"=0.0, "Color Box"=0}, {"Mean"=0.0, " Std"=0.0, "Color Box"=0}, {"Mean"=0.0, " Std"=0.0, "Color Box"=0}, {"Mean"=0.0, " Std"=0.0, "Color Box"=0}, {"Mean"=0.0, " Std"=0.0, "Color Box"=0}, {"Mean"=0.0, " Std"=0.0, "Color Box"=0}, {"Mean"=0.0, " Std"=0.0, "Color Box"=0}, {"Mean"=0.0, " Std"=0.0, "Color Box"=0}, {"Mean"=0.0, " Std"=0.0, "Color Box"=0}, {"Mean"=0.0, " Std"=0.0, "Color Box"=0}, {"Mean"=0.0, " Std"=0.0, "Color Box"=0}, {"Mean"=0.0, " Std"=0.0, "Color Box"=0}, {"Mean"=0.0, " Std"=0.0, "Color Box"=0}, {"Mean"=0.0, " Std"=0.0, "Color Box"=0}, {"Mean"=0.0, " Std"=0.0, "Color Box"=0}, {"Mean"=0.0, " Std"=0.0, "Color Box"=0}, {"Mean"=0.0, " Std"=0.0, "Color Box"=0}, {"Mean"=0.0, " Std"=0.0, "Color Box"=0}, {"Mean"=0.0, " Std"=0.0, "Color Box"=0}, {"Mean"=0.0, " Std"=0.0, "Color Box"=0}, {"Mean"=0.0, " Std"=0.0, "Color Box"=0}, {"Mean"=0.0, " Std"=0.0, "Color Box"=0}, {"Mean"=0.0, " Std"=0.0, "Color Box"=0}, {"Mean"=0.0, " Std"=0.0, "Color Box"=0}, {"Mean"=0.0, " Std"=0.0, "Color Box"=0}, {"Mean"=0.0, " Std"=0.0, "Color Box"=0}, {"Mean"=0.0, " Std"=0.0, "Color Box"=0}, {"Mean"=0.0, " Std"=0.0, "Color Box"=0}, {"Mean"=0.0, " Std"=0.0, "Color Box"=0}, {"Mean"=0.0, " Std"=0.0, "Color Box"=0}, {"Mean"=0.0, " Std"=0.0, "Color Box"=0}, {"Mean"=0.0, " Std"=0.0, "Color Box"=0}, {"Mean"=0.0, " Std"=0.0, "Color Box"=0}, {"Mean"=0.0, " Std"=0.0, "Color Box"=0}, {"Mean"=0.0, " Std"=0.0, "Color Box"=0}, {"Mean"=0.0, " Std"=0.0, "Color Box"=0}, {"Mean"=0.0, " Std"=0.0, "Color Box"=0}, {"Mean"=0.0, " Std"=0.0, "Color Box"=0}, {"Mean"=0.0, " Std"=0.0, "Color Box"=0}, {"Mean"=0.0, " Std"=0.0, "Color Box"=0}, {"Mean"=0.0, " Std"=0.0, "Color Box"=0}, {"Mean"=0.0, " Std"=0.0, "Color Box"=0}, {"Mean"=0.0, " Std"=0.0, "Color Box"=0}, {"Mean"=0.0, " Std"=0.0, "Color Box"=0}, {"Mean"=0.0, " Std"=0.0, "Color Box"=0}, {"Mean"=0.0, " Std"=0.0, "Color Box"=0}, {"Mean"=0.0, " Std"=0.0, "Color Box"=0}, {"Mean"=0.0, " Std"=0.0, "Color Box"=0}, {"Mean"=0.0, " Std"=0.0, "Color Box"=0}, {"Mean"=0.0, " Std"=0.0, "Color Box"=0}, {"Mean"=0.0, " Std"=0.0, "Color Box"=0}, {"Mean"=0.0, " Std"=0.0, "Color Box"=0}, {"Mean"=0.0, " Std"=0.0, "Color Box"=0}, {"Mean"=0.0, " Std"=0.0, "Color Box"=0}, {"Mean"=0.0, " Std"=0.0, "Color Box"=0}, {"Mean"=0.0, " Std"=0.0, "Color Box"=0}, {"Mean"=0.0, " Std"=0.0, "Color Box"=0}, {"Mean"=0.0, " Std"=0.0, "Color Box"=0}, {"Mean"=0.0, " Std"=0.0, "Color Box"=0}, {"Mean"=0.0, " Std"=0.0, "Color Box"=0}, {"Mean"=0.0, " Std"=0.0, "Color Box"=0}, {"Mean"=0.0, " Std"=0.0, "Color Box"=0}, {"Mean"=0.0, " Std"=0.0, "Color Box"=0}, {"Mean"=0.0, " Std"=0.0, "Color Box"=0}, {"Mean"=0.0, " Std"=0.0, "Color Box"=0}, {"Mean"=0.0, " Std"=0.0, "Color Box"=0}, {"Mean"=0.0, " Std"=0.0, "Color Box"=0}, {"Mean"=0.0, " Std"=0.0, "Color Box"=0}, {"Mean"=0.0, " Std"=0.0, "Color Box"=0}, {"Mean"=0.0, " Std"=0.0, "Color Box"=0}, {"Mean"=0.0, " Std"=0.0, "Color Box"=0}, {"Mean"=0.0, " Std"=0.0, "Color Box"=0}, {"Mean"=0.0, " Std"=0.0, "Color Box"=0}, {"Mean"=0.0, " Std"=0.0, "Color Box"=0}, {"Mean"=0.0, " Std"=0.0, "Color Box"=0}, {"Mean"=0.0, " Std"=0.0, "Color Box"=0}, {"Mean"=0.0, " Std"=0.0, "Color Box"=0}, {"Mean"=0.0, " Std"=0.0, "Color Box"=0}, {"Mean"=0.0, " Std"=0.0, "Color Box"=0}, {"Mean"=0.0, " Std"=0.0, "Color Box"=0}, {"Mean"=0.0, " Std"=0.0, "Color Box"=0}, {"Mean"=0.0, " Std"=0.0, "Color Box"=0}, {"Mean"=0.0, " Std"=0.0, "Color Box"=0}, {"Mean"=0.0, " Std"=0.0, "Color Box"=0}, {"Mean"=0.0, " Std"=0.0, "Color Box"=0}, {"Mean"=0.0, " Std"=0.0, "Color Box"=0}, {"Mean"=0.0, " Std"=0.0, "Color Box"=0}, {"Mean"=0.0, " Std"=0.0, "Color Box"=0}, {"Mean"=0.0, " Std"=0.0, "Color Box"=0}, {"Mean"=0.0, " Std"=0.0, "Color Box"=0}, {"Mean"=0.0, " Std"=0.0, "Color Box"=0}, {"Mean"=0.0, " Std"=0.0, "Color Box"=0}, {"Mean"=0.0, " Std"=0.0, "Color Box"=0}, {"Mean"=0.0, " Std"=0.0, "Color Box"=0}, {"Mean"=0.0, " Std"=0.0, "Color Box"=0}, {"Mean"=0.0, " Std"=0.0, "Color Box"=0}, {"Mean"=0.0, " Std"=0.0, "Color Box"=0}, {"Mean"=0.0, " Std"=0.0, "Color Box"=0}, {"Mean"=0.0, " Std"=0.0, "Color Box"=0}, {"Mean"=0.0, " Std"=0.0, "Color Box"=0}, {"Mean"=0.0, " Std"=0.0, "Color Box"=0}, {"Mean"=0.0, " Std"=0.0, "Color Box"=0}, {"Mean"=0.0, " Std"=0.0, "Color Box"=0}, {"Mean"=0.0, " Std"=0.0, "Color Box"=0}, {"Mean"=0.0, " Std"=0.0, "Color Box"=0}, {"Mean"=0.0, " Std"=0.0, "Color Box"=0}, {"Mean"=0.0, " Std"=0.0, "Color Box"=0}, {"Mean"=0.0, " Std"=0.0, "Color Box"=0}, {"Mean"=0.0, " Std"=0.0, "Color Box"=0}, {"Mean"=0.0, " Std"=0.0, "Color Box"=0}, {"Mean"=0.0, " Std"=0.0, "Color Box"=0}, {"Mean"=0.0, " Std"=0.0, "Color Box"=0}, {"Mean"=0.0, " Std"=0.0, "Color Box"=0}, {"Mean"=0.0, " Std"=0.0, "Color Box"=0}, {"Mean"=0.0, " Std"=0.0, "Color Box"=0}, {"Mean"=0.0, " Std"=0.0, "Color Box"=0}, {"Mean"=0.0, " Std"=0.0, "Color Box"=0}, {"Mean"=0.0, " Std"=0.0, "Color Box"=0}, {"Mean"=0.0, " Std"=0.0, "Color Box"=0}, {"Mean"=0.0, " Std"=0.0, "Color Box"=0}, {"Mean"=0.0, " Std"=0.0, "Color Box"=0}, {"Mean"=0.0, " Std"=0.0, "Color Box"=0}, {"Mean"=0.0, " Std"=0.0, "Color Box"=0}, {"Mean"=0.0, " Std"=0.0, "Color Box"=0}, {"Mean"=0.0, " Std"=0.0, "Color Box"=0}, {"Mean"=0.0, " Std"=0.0, "Color Box"=0}, {"Mean"=0.0, " Std"=0.0, "Color Box"=0}, {"Mean"=0.0, " Std"=0.0, "Color Box"=0}, {"Mean"=0.0, " Std"=0.0, "Color Box"=0}, {"Mean"=0.0, " Std"=0.0, "Color Box"=0}, {"Mean"=0.0, " Std"=0.0, "Color Box"=0}, {"Mean"=0.0, " Std"=0.0, "Color Box"=0}, {"Mean"=0.0, " Std"=0.0, "Color Box"=0}, {"Mean"=0.0, " Std"=0.0, "Color Box"=0}, {"Mean"=0.0, " Std"=0.0, "Color Box"=0}, {"Mean"=0.0, " Std"=0.0, "Color Box"=0}, {"Mean"=0.0, " Std"=0.0, "Color Box"=0}, {"Mean"=0.0, " Std"=0.0, "Color Box"=0}, {"Mean"=0.0, " Std"=0.0, "Color Box"=0}, {"Mean"=0.0, " Std"=0.0, "Color Box"=0}, {"Mean"=0.0, " Std"=0.0, "Color Box"=0}, {"Mean"=0.0, " Std"=0.0, "Color Box"=0}, {"Mean"=0.0, " Std"=0.0, "Color Box"=0}, {"Mean"=0.0, " Std"=0.0, "Color Box"=0}, {"Mean"=0.0, " Std"=0.0, "Color Box"=0}, {"Mean"=0.0, " Std"=0.0, "Color Box"=0}, {"Mean"=0.0, " Std"=0.0, "Color Box"=0}, {"Mean"=0.0, " Std"=0.0, "Color Box"=0}, {"Mean"=0.0, " Std"=0.0, "Color Box"=0}, {"Mean"=0.0, " Std"=0.0, "Color Box"=0}, {"Mean"=0.0, " Std"=0.0, "Color Box"=0}, {"Mean"=0.0, " Std"=0.0, "Color Box"=0}, {"Mean"=0.0, " Std"=0.0, "Color Box"=0}, {"Mean"=0.0, " Std"=0.0, "Color Box"=0}, {"Mean"=0.0, " Std"=0.0, "Color Box"=0}, {"Mean"=0.0, " Std"=0.0, "Color Box"=0}, {"Mean"=0.0, " Std"=0.0, "Color Box"=0}, {"Mean"=0.0, " Std"=0.0, "Color Box"=0}, {"Mean"=0.0, " Std"=0.0, "Color Box"=0}, {"Mean"=0.0, " Std"=0.0, "Color Box"=0}, {"Mean"=0.0, " Std"=0.0, "Color Box"=0}, {"Mean"=0.0, " Std"=0.0, "Color Box"=0}, {"Mean"=0.0, " Std"=0.0, "Color Box"=0}, {"Mean"=0.0, " Std"=0.0, "Color Box"=0}, {"Mean"=0.0, " Std"=0.0, "Color Box"=0}, {"Mean"=0.0, " Std"=0.0, "Color Box"=0}, {"Mean"=0.0, " Std"=0.0, "Color Box"=0}, {"Mean"=0.0, " Std"=0.0, "Color Box"=0}, {"Mean"=0.0, " Std"=0.0, "Color Box"=0}, {"Mean"=0.0, " Std"=0.0, "Color Box"=0}, {"Mean"=0.0, " Std"=0.0, "Color Box"=0}, {"Mean"=0.0, " Std"=0.0, "Color Box"=0}, {"Mean"=0.0, " Std"=0.0, "Color Box"=0}, {"Mean"=0.0, " Std"=0.0, "Color Box"=0}, {"Mean"=0.0, " Std"=0.0, "Color Box"=0}, {"Mean"=0.0, " Std"=0.0, "Color Box"=0}, {"Mean"=0.0, " Std"=0.0, "Color Box"=0}, {"Mean"=0.0, " Std"=0.0, "Color Box"=0}, {"Mean"=0.0, " Std"=0.0, "Color Box"=0}, {"Mean"=0.0, " Std"=0.0, "Color Box"=0}, {"Mean"=0.0, " Std"=0.0, "Color Box"=0}, {"Mean"=0.0, " Std"=0.0, "Color Box"=0}, {"Mean"=0.0, " Std"=0.0, "Color Box"=0}, {"Mean"=0.0, " Std"=0.0, "Color Box"=0}, {"Mean"=0.0, " Std"=0.0, "Color Box"=0}, {"Mean"=0.0, " Std"=0.0, "Color Box"=0}, {"Mean"=0.0, " Std"=0.0, "Color Box"=0}, {"Mean"=0.0, " Std"=0.0, "Color Box"=0}, {"Mean"=0.0, " Std"=0.0, "Color Box"=0}, {"Mean"=0.0, " Std"=0.0, "Color Box"=0}, {"Mean"=0.0, " Std"=0.0, "Color Box"=0}, {"Mean"=0.0, " Std"=0.0, "Color Box"=0}, {"Mean"=0.0, " Std"=0.0, "Color Box"=0}, {"Mean"=0.0, " Std"=0.0, "Color Box"=0}, {"Mean"=0.0, " Std"=0.0, "Color Box"=0}, {"Mean"=0.0, " Std"=0.0, "Color Box"=0}, {"Mean"=0.0, " Std"=0.0, "Color Box"=0}, {"Mean"=0.0, " Std"=0.0, "Color Box"=0}, {"Mean"=0.0, " Std"=0.0, "Color Box"=0}, {"Mean"=0.0, " Std"=0.0, "Color Box"=0}, {"Mean"=0.0, " Std"=0.0, "Color Box"=0}, {"Mean"=0.0, " Std"=0.0, "Color Box"=0}, {"Mean"=0.0, " Std"=0.0, "Color Box"=0}, {"Mean"=0.0, " Std"=0.0, "Color Box"=0}, {"Mean"=0.0, " Std"=0.0, "Color Box"=0}, {"Mean"=0.0, " Std"=0.0, "Color Box"=0}, {"Mean"=0.0, " Std"=0.0, "Color Box"=0}, {"Mean"=0.0, " Std"=0.0, "Color Box"=0}, {"Mean"=0.0, " Std"=0.0, "Color Box"=0}, {"Mean"=0.0, " Std"=0.0, "Color Box"=0}, {"Mean"=0.0, " Std"=0.0, "Color Box"=0}, {"Mean"=0.0, " Std"=0.0, "Color Box"=0}, {"Mean"=0.0, " Std"=0.0, "Color Box"=0}, {"Mean"=0.0, " Std"=0.0, "Color Box"=0}, {"Mean"=0.0, " Std"=0.0, "Color Box"=0}, {"Mean"=0.0, " Std"=0.0, "Color Box"=0}, {"Mean"=0.0, " Std"=0.0, "Color Box"=0}, {"Mean"=0.0, " Std"=0.0, "Color Box"=0}, {"Mean"=0.0, " Std"=0.0, "Color Box"=0}, {"Mean"=0.0, " Std"=0.0, "Color Box"=0}, {"Mean"=0.0, " Std"=0.0, "Color Box"=0}, {"Mean"=0.0, " Std"=0.0, "Color Box"=0}, {"Mean"=0.0, " Std"=0.0, "Color Box"=0}, {"Mean"=0.0, " Std"=0.0, "Color Box"=0}, {"Mean"=0.0, " Std"=0.0, "Color Box"=0}, {"Mean"=0.0, " Std"=0.0, "Color Box"=0}, {"Mean"=0.0, " Std"=0.0, "Color Box"=0}, {"Mean"=0.0, " Std"=0.0, "Color Box"=0}, {"Mean"=0.0, " Std"=0.0, "Color Box"=0}, {"Mean"=0.0, " Std"=0.0, "Color Box"=0}, {"Mean"=0.0, " Std"=0.0, "Color Box"=0}, {"Mean"=0.0, " Std"=0.0, "Color Box"=0}, {"Mean"=0.0, " Std"=0.0, "Color Box"=0}, {"Mean"=0.0, " Std"=0.0, "Color Box"=0}, {"Mean"=0.0, " Std"=0.0, "Color Box"=0}, {"Mean"=0.0, " Std"=0.0, "Color Box"=0}, {"Mean"=0.0, " Std"=0.0, "Color Box"=0}, {"Mean"=0.0, " Std"=0.0, "Color Box"=0}, {"Mean"=0.0, " Std"=0.0, "Color Box"=0}, {"Mean"=0.0, " Std"=0.0, "Color Box"=0}, {"Mean"=0.0, " Std"=0.0, "Color Box"=0}, {"Mean"=0.0, " Std"=0.0, "Color Box"=0}, {"Mean"=0.0, " Std"=0.0, "Color Box"=0}, {"Mean"=0.0, " Std"=0.0, "Color Box"=0}, {"Mean"=0.0, " Std"=0.0, "Color Box"=0}, {"Mean"=0.0, " Std"=0.0, "Color Box"=0}, {"Mean"=0.0, " Std"=0.0, "Color Box"=0}, {"Mean"=0.0, " Std"=0.0, "Color Box"=0}, {"Mean"=0.0, " Std"=0.0, "Color Box"=0}, {"Mean"=0.0, " Std"=0.0, "Color Box"=0}, {"Mean"=0.0, " Std"=0.0, "Color Box"=0}, {"Mean"=0.0, " Std"=0.0, "Color Box"=0}, {"Mean"=0.0, " Std"=0.0, "Color Box"=0}, {"Mean"=0.0, " Std"=0.0, "Color Box"=0}, {"Mean"=0.0, " Std"=0.0, "Color Box"=0}, {"Mean"=0.0, " Std"=0.0, "Color Box"=0}, {"Mean"=0.0, " Std"=0.0, "Color Box"=0}, {"Mean"=0.0, " Std"=0.0, "Color Box"=0}, {"Mean"=0.0, " Std"=0.0, "Color Box"=0}, {"Mean"=0.0, " Std"=0.0, "Color Box"=0}, {"Mean"=0.0, " Std"=0.0, "Color Box"=0}, {"Mean"=0.0, " Std"=0.0, "Color Box"=0}, {"Mean"=0.0, " Std"=0.0, "Color Box"=0}, {"Mean"=0.0, " Std"=0.0, "Color Box"=0}, {"Mean"=0.0, " Std"=0.0, "Color Box"=0}, {"Mean"=0.0, " Std"=0.0, "Color Box"=0}, {"Mean"=0.0, " Std"=0.0, "Color Box"=0}, {"Mean"=0.0, " Std"=0.0, "Color Box"=0}, {"Mean"=0.0, " Std"=0.0, "Color Box"=0}, {"Mean"=0.0, " Std"=0.0, "Color Box"=0}, {"Mean"=0.0, " Std"=0.0, "Color Box"=0}, {"Mean"=0.0, " Std"=0.0, "Color Box"=0}, {"Mean"=0.0, " Std"=0.0, "Color Box"=0}, {"Mean"=0.0, " Std"=0.0, "Color Box"=0}, {"Mean"=0.0, " Std"=0.0, "Color Box"=0}, {"Mean"=0.0, " Std"=0.0, "Color Box"=0}, {"Mean"=0.0, " Std"=0.0, "Color Box"=0}, {"Mean"=0.0, " Std"=0.0, "Color Box"=0}, {"Mean"=0.0, " Std"=0.0, "Color Box"=0}, {"Mean"=0.0, " Std"=0.0, "Color Box"=0}, {"Mean"=0.0, " Std"=0.0, "Color Box"=0}, {"Mean"=0.0, " Std"=0.0, "Color Box"=0}, {"Mean"=0.0, " Std"=0.0, "Color Box"=0}, {"Mean"=0.0, " Std"=0.0, "Color Box"=0}, {"Mean"=0.0, " Std"=0.0, "Color Box"=0}, {"Mean"=0.0, " Std"=0.0, "Color Box"=0}, {"Mean"=0.0, " Std"=0.0, "Color Box"=0}, {"Mean"=0.0, " Std"=0.0, "Color Box"=0}, {"Mean"=0.0, " Std"=0.0, "Color Box"=0}, {"Mean"=0.0, " Std"=0.0, "Color Box"=0}, {"Mean"=0.0, " Std"=0.0, "Color Box"=0}, {"Mean"=0.0, " Std"=0.0, "Color Box"=0}, {"Mean"=0.0, " Std"=0.0, "Color Box"=0}, {"Mean"=0.0, " Std"=0.0, "Color Box"=0}, {"Mean"=0.0, " Std"=0.0, "Color Box"=0}, {"Mean"=0.0, " Std"=0.0, "Color Box"=0}, {"Mean"=0.0, " Std"=0.0, "Color Box"=0}, {"Mean"=0.0, " Std"=0.0, "Color Box"=0}, {"Mean"=0.0, " Std"=0.0, "Color Box"=0}, {"Mean"=0.0, " Std"=0.0, "Color Box"=0}, {"Mean"=0.0, " Std"=0.0, "Color Box"=0}, {"Mean"=0.0, " Std"=0.0, "Color Box"=0}, {"Mean"=0.0, " Std"=0.0, "Color Box"=0}, {"Mean"=0.0, " Std"=0.0, "Color Box"=0}, {"Mean"=0.0, " Std"=0.0, "Color Box"=0}, {"Mean"=0.0, " Std"=0.0, "Color Box"=0}, {"Mean"=0.0, " Std"=0.0, "Color Box"=0}, {"Mean"=0.0, " Std"=0.0, "Color Box"=0}, {"Mean"=0.0, " Std"=0.0, "Color Box"=0}, {"Mean"=0.0, " Std"=0.0, "Color Box"=0}, {"Mean"=0.0, " Std"=0.0, "Color Box"=0}, {"Mean"=0.0, " Std"=0.0, "Color Box"=0}, {"Mean"=0.0, " Std"=0.0, "Color Box"=0}, {"Mean"=0.0, " Std"=0.0, "Color Box"=0}, {"Mean"=0.0, " Std"=0.0, "Color Box"=0}, {"Mean"=0.0, " Std"=0.0, "Color Box"=0}, {"Mean"=0.0, " Std"=0.0, "Color Box"=0}, {"Mean"=0.0, " Std"=0.0, "Color Box"=0}, {"Mean"=0.0, " Std"=0.0, "Color Box"=0}, {"Mean"=0.0, " Std"=0.0, "Color Box"=0}, {"Mean"=0.0, " Std"=0.0, "Color Box"=0}, {"Mean"=0.0, " Std"=0.0, "Color Box"=0}, {"Mean"=0.0, " Std"=0.0, "Color Box"=0}, {"Mean"=0.0, " Std"=0.0, "Color Box"=0}, {"Mean"=0.0, " Std"=0.0, "Color Box"=0}, {"Mean"=0.0, " Std"=0.0, "Color Box"=0}, {"Mean"=0.0, " Std"=0.0, "Color Box"=0}, {"Mean"=0.0, " Std"=0.0, "Color Box"=0}, {"Mean"=0.0, " Std"=0.0, "Color Box"=0}, {"Mean"=0.0, " Std"=0.0, "Color Box"=0}, {"Mean"=0.0, " Std"=0.0, "Color Box"=0}, {"Mean"=0.0, " Std"=0.0, "Color Box"=0}, {"Mean"=0.0, " Std"=0.0, "Color Box"=0}, {"Mean"=0.0, " Std"=0.0, "Color Box"=0}, {"Mean"=0.0, " Std"=0.0, "Color Box"=0}, {"Mean"=0.0, " Std"=0.0, "Color Box"=0}, {"Mean"=0.0, " Std"=0.0, "Color Box"=0}, {"Mean"=0.0, " Std"=0.0, "Color Box"=0}, {"Mean"=0.0, " Std"=0.0, "Color Box"=0}, {"Mean"=0.0, " Std"=0.0, "Color Box"=0}, {"Mean"=0.0, " Std"=0.0, "Color Box"=0}, {"Mean"=0.0, " Std"=0.0, "Color Box"=0}, {"Mean"=0.0, " Std"=0.0, "Color Box"=0}, {"Mean"=0.0, " Std"=0.0, "Color Box"=0}, {"Mean"=0.0, " Std"=0.0, "Color Box"=0}, {"Mean"=0.0, " Std"=0.0, "Color Box"=0}, {"Mean"=0.0, " Std"=0.0, "Color Box"=0}, {"Mean"=0.0, " Std"=0.0, "Color Box"=0}, {"Mean"=0.0, " Std"=0.0, "Color Box"=0}, {"Mean"=0.0, " Std"=0.0, "Color Box"=0}, {"Mean"=0.0, " Std"=0.0, "Color Box"=0}, {"Mean"=0.0, " Std"=0.0, "Color Box"=0}, {"Mean"=0.0, " Std"=0.0, "Color Box"=0}, {"Mean"=0.0, " Std"=0.0, "Color Box"=0}, {"Mean"=0.0, " Std"=0.0, "Color Box"=0}, {"Mean"=0.0, " Std"=0.0, "Color Box"=0}, {"Mean"=0.0, " Std"=0.0, "Color Box"=0}, {"Mean"=0.0, " Std"=0.0, "Color Box"=0}, {"Mean"=0.0, " Std"=0.0, "Color Box"=0}, {"Mean"=0.0, " Std"=0.0, "Color Box"=0}, {"Mean"=0.0, " Std"=0.0, "Color Box"=0}, {"Mean"=0.0, " Std"=0.0, "Color Box"=0}, {"Mean"=0.0, " Std"=0.0, "Color Box"=0}, {"Mean"=0.0, " Std"=0.0, "Color Box"=0}, {"Mean"=0.0, " Std"=0.0, "Color Box"=0}, {"Mean"=0.0, " Std"=0.0, "Color Box"=0}, {"Mean"=0.0, " Std"=0.0, "Color Box"=0}, {"Mean"=0.0, " Std"=0.0, "Color Box"=0}, {"Mean"=0.0, " Std"=0.0, "Color Box"=0}, {"Mean"=0.0, " Std"=0.0, "Color Box"=0}, {"Mean"=0.0, " Std"=0.0, "Color Box"=0}, {"Mean"=0.0, " Std"=0.0, "Color Box"=0}, {"Mean"=0.0, " Std"=0.0, "Color Box"=0}, {"Mean"=0.0, " Std"=0.0, "Color Box"=0}, {"Mean"=0.0, " Std"=0.0, "Color Box"=0}, {"Mean"=0.0, " Std"=0.0, "Color Box"=0}, {"Mean"=0.0, " Std"=0.0, "Color Box"=0}, {"Mean"=0.0, " Std"=0.0, "Color Box"=0}, {"Mean"=0.0, " Std"=0.0, "Color Box"=0}, {"Mean"=0.0, " Std"=0.0, "Color Box"=0}, {"Mean"=0.0, " Std"=0.0, "Color Box"=0}, {"Mean"=0.0, " Std"=0.0, "Color Box"=0}, {"Mean"=0.0, " Std"=0.0, "Color Box"=0}, {"Mean"=0.0, " Std"=0.0, "Color Box"=0}, {"Mean"=0.0, " Std"=0.0, "Color Box"=0}, {"Mean"=0.0, " Std"=0.0, "Color Box"=0}, {"Mean"=0.0, " Std"=0.0, "Color Box"=0}, {"Mean"=0.0, " Std"=0.0, "Color Box"=0}, {"Mean"=0.0, " Std"=0.0, "Color Box"=0}, {"Mean"=0.0, " Std"=0.0, "Color Box"=0}, {"Mean"=0.0, " Std"=0.0, "Color Box"=0}, {"Mean"=0.0, " Std"=0.0, "Color Box"=0}, {"Mean"=0.0, " Std"=0.0, "Color Box"=0}, {"Mean"=0.0, " Std"=0.0, "Color Box"=0}, {"Mean"=0.0, " Std"=0.0, "Color Box"=0}, {"Mean"=0.0, " Std"=0.0, "Color Box"=0}, {"Mean"=0.0, " Std"=0.0, "Color Box"=0}, {"Mean"=0.0, " Std"=0.0, "Color Box"=0}, {"Mean"=0.0, " Std"=0.0, "Color Box"=0}, {"Mean"=0.0, " Std"=0.0, "Color Box"=0}, {"Mean"=0.0, " Std"=0.0, "Color Box"=0}, {"Mean"=0.0, " Std"=0.0, "Color Box"=0}, {"Mean"=0.0, " Std"=0.0, "Color Box"=0}, {"Mean"=0.0, " Std"=0.0, "Color Box"=0}, {"Mean"=0.0, " Std"=0.0, "Color Box"=0}, {"Mean"=0.0, " Std"=0.0, "Color Box"=0}, {"Mean"=0.0, " Std"=0.0, "Color Box"=0}, {"Mean"=0.0, " Std"=0.0, "Color Box"=0}, {"Mean"=0.0, " Std"=0.0, "Color Box"=0}, {"Mean"=0.0, " Std"=0.0, "Color Box"=0}, {"Mean"=0.0, " Std"=0.0, "Color Box"=0}, {"Mean"=0.0, " Std"=0.0, "Color Box"=0}, {"Mean"=0.0, " Std"=0.0, "Color Box"=0}, {"Mean"=0.0, " Std"=0.0, "Color Box"=0}, {"Mean"=0.0, " Std"=0.0, "Color Box"=0}, {"Mean"=0.0, " Std"=0.0, "Color Box"=0}, {"Mean"=0.0, " Std"=0.0, "Color Box"=0}, {"Mean"=0.0, " Std"=0.0, "Color Box"=0}, {"Mean"=0.0, " Std"=0.0, "Color Box"=0}, {"Mean"=0.0, " Std"=0.0, "Color Box"=0}, {"Mean"=0.0, " Std"=0.0, "Color Box"=0}, {"Mean"=0.0, " Std"=0.0, "Color Box"=0}, {"Mean"=0.0, " Std"=0.0, "Color Box"=0}, {"Mean"=0.0, " Std"=0.0, "Color Box"=0}, {"Mean"=0.0, " Std"=0.0, "Color Box"=0}, {"Mean"=0.0, " Std"=0.0, "Color Box"=0}, {"Mean"=0.0, " Std"=0.0, "Color Box"=0}, {"Mean"=0.0, " Std"=0.0, "Color Box"=0}, {"Mean"=0.0, " Std"=0.0, "Color Box"=0}, {"Mean"=0.0, " Std"=0.0, "Color Box"=0}, {"Mean"=0.0, " Std"=0.0, "Color Box"=0}, {"Mean"=0.0, " Std"=0.0, "Color Box"=0}, {"Mean"=0.0, " Std"=0.0, "Color Box"=0}, {"Mean"=0.0, " Std"=0.0, "Color Box"=0}, {"Mean"=0.0, " Std"=0.0, "Color Box"=0}, {"Mean"=0.0, " Std"=0.0, "Color Box"=0}, {"Mean"=0.0, " Std"=0.0, "Color Box"=0}, {"Mean"=0.0, " Std"=0.0, "Color Box"=0}, {"Mean"=0.0, " Std"=0.0, "Color Box"=0}, {"Mean"=0.0, " Std"=0.0, "Color Box"=0}, {"Mean"=0.0, " Std"=0.0, "Color Box"=0}, {"Mean"=0.0, " Std"=0.0, "Color Box"=0}, {"Mean"=0.0, " Std"=0.0, "Color Box"=0}, {"Mean"=0.0, " Std"=0.0, "Color Box"=0}, {"Mean"=0.0, " Std"=0.0, "Color Box"=0}, {"Mean"=0.0, " Std"=0.0, "Color Box"=0}, {"Mean"=0.0, " Std"=0.0, "Color Box"=0}, {"Mean"=0.0, " Std"=0.0, "Color Box"=0}, {"Mean"=0.0, " Std"=0.0, "Color Box"=0}, {"Mean"=0.0, " Std"=0.0, "Color Box"=0}, {"Mean"=0.0, " Std"=0.0, "Color Box"=0}, {"Mean"=0.0, " Std"=0.0, "Color Box"=0}, {"Mean"=0.0, " Std"=0.0, "Color Box"=0}, {"Mean"=0.0, " Std"=0.0, "Color Box"=0}, {"Mean"=0.0, " Std"=0.0, "Color Box"=0}, {"Mean"=0.0, " Std"=0.0, "Color Box"=0}, {"Mean"=0.0, " Std"=0.0, "Color Box"=0}, {"Mean"=0.0, " Std"=0.0, "Color Box"=0}, {"Mean"=0.0, " Std"=0.0, "Color Box"=0}, {"Mean"=0.0, " Std"=0.0, "Color Box"=0}, {"Mean"=0.0, " Std"=0.0, "Color Box"=0}, {"Mean"=0.0, " Std"=0.0, "Color Box"=0}, {"Mean"=0.0, " Std"=0.0, "Color Box"=0}, {"Mean"=0.0, " Std"=0.0, "Color Box"=0}, {"Mean"=0.0, " Std"=0.0, "Color Box"=0}, {"Mean"=0.0, " Std"=0.0, "Color Box"=0}, {"Mean"=0.0, " Std"=0.0, "Color Box"=0}, {"Mean"=0.0, " Std"=0.0, "Color Box"=0}, {"Mean"=0.0, " Std"=0.0, "Color Box"=0}, {"Mean"=0.0, " Std"=0.0, "Color Box"=0}, {"Mean"=0.0, " Std"=0.0, "Color Box"=0}, {"Mean"=0.0, " Std"=0.0, "Color Box"=0}, {"Mean"=0.0, " Std"=0.0, "Color Box"=0}, {"Mean"=0.0, " Std"=0.0, "Color Box"=0}, {"Mean"=0.0, " Std"=0.0, "Color Box"=0}, {"Mean"=0.0, " Std"=0.0, "Color Box"=0}, {"Mean"=0.0, " Std"=0.0, "Color Box"=0}, {"Mean"=0.0, " Std"=0.0, "Color Box"=0}, {"Mean"=0.0, " Std"=0.0, "Color Box"=0}, {"Mean"=0.0, " Std"=0.0, "Color Box"=0}, {"Mean"=0.0, " Std"=0.0, "Color Box"=0}, {"Mean"=0.0, " Std"=0.0, "Color Box"=0}, {"Mean"=0.0, " Std"=0.0, "Color Box"=0}, {"Mean"=0.0, " Std"=0.0, "Color Box"=0}, {"Mean"=0.0, " Std"=0.0, "Color Box"=0}, {"Mean"=0.0, " Std"=0.0, "Color Box"=0}, {"Mean"=0.0, " Std"=0.0, "Color Box"=0}, {"Mean"=0.0, " Std"=0.0, "Color Box"=0}, {"Mean"=0.0, " Std"=0.0, "Color Box"=0}, {"Mean"=0.0, " Std"=0.0, "Color Box"=0}]  # Test Data Array
        w122 = T9 {"Current VI Reference"=refnum, "Close Panel on Exit?"=FALSE}  # Core
        # "MW100 References"
        # "EQUIP VISA References"
        n44 = call "HEWH Calibration File Check.vi"("error in (no error)"=w114, "Calibration Path"="Calibration Path") -> ("error out"=w112:errorcluster, "Calibration Path"=→"Calibration File Path":path, "Calibration File Array"=→"Calibration File Array":dbl[][], "Complete File?"=→"Calibration File?":bool)  [unwired: 6 in]
        n45 = call "HEWH Channel Test Labels.vi"("RunTime"=TRUE ("Stop")) -> ("Channel List"=w111:string)  [unwired: 12 in, 2 out]
        n46 = call "HEWH Initialize Equipmet.vi"("Error In"=w112, "Core HEWH Data"=w111, "Test Fixture Hardware"="Equipment") -> ("Error Out"=w110:errorcluster, "HEWH Power"=w120:bool)  [unwired: 7 in]
        n47 = Bundle("Core"=w122, "Num Samples"="Num Samples", "HEWH Power"=w120, "Test Data Array"=w119, "Channel List"=w111) -> (w123:T8)  [unwired: 1 in]
        n48 = call <vilib>:"Add State(s) to Queue__jki_lib_state_machine.vi"("State(s) in (\"\")"=w125) -> ("States Out"=w124:string)  [unwired: 14 in]
      }
      frame "Get Agilent Scan List" {
        n49 = call "HEWH Channel Test Labels.vi"("RunTime"=FALSE) -> ("Agilent Cluster Array"=w130:T10[], "Channel List"=w128:string)  [unwired: 12 in, 1 out]
        n50 = String Length(string=w128) -> (length=w126:i32)
        n51 = Greater Than 0?(x=w126) -> (x > 0?=w129:bool)
        "Use Agilent?" <- w129
        n52 = Bundle By Name("Agilent Cluster Array"=w130, "Agilent Channel List"=w128, "Use Agilent?"=w129) -> ()  [unwired: 1 in, 1 out]
        n53 = call <vilib>:"Add State(s) to Queue__jki_lib_state_machine.vi"("State(s) in (\"\")"=w133) -> ("States Out"=w132:string)  [unwired: 14 in]
      }
      frame "Initialize Equipment" {
        # "Give it a second to make sure\neverything is setup."
        n54 = Unbundle By Name() -> (w139:T25, "User Controls.Use Agilent?"=w140, "Equipment VISA"=w137, "FileInit Cluster.Agilent Channel List"=w138, "Power Analyzer"=w141)
        n55 = call "HEWH Initialize Equipmet.vi"("Use Agilent?"=w140, "Pressurize Tank"=w141, "Core HEWH Data"=w138, "Test Fixture Hardware"=w137) -> ()  [unwired: 6 in, 2 out]
        n56 = call <vilib>:"Add State(s) to Queue__jki_lib_state_machine.vi"("State(s) in (\"\")"=w143) -> ("States Out"=w142:string)  [unwired: 14 in]
        n57 = call "UTILITY Delay mS.vi"("Error In"=w135, "milliseconds to wait"=u32 1000) -> ("Error Out"=w134:errorcluster)  [unwired: 13 in]
      }
      frame "Data: Cleanup" {
        n58 = Unbundle By Name(w147) -> ("Core.Current VI Reference"=w149:refnum<vi>, "Equipment Out"=w146)
        n59 = call "HEWH Close Equipmet.vi"("Error In"=w144, "Test Fixture Hardware In"=w146) -> ("Error Out"=w145:errorcluster)  [unwired: 8 in, 1 out]
        n60 = Close Reference(reference=w149, error in (no error)=w145) -> (error out=w148:errorcluster)
        n61 = call <vilib>:"Add State(s) to Queue__jki_lib_state_machine.vi"("State(s) in (\"\")"=w151) -> ("States Out"=w150:string)  [unwired: 14 in]
      }
      frame "---------- UI ----------" {
        n62 = call <vilib>:"Add State(s) to Queue__jki_lib_state_machine.vi"("State(s) in (\"\")"=w155) -> ("States Out"=w154:string)  [unwired: 14 in]
      }
      frame "UI: Initialize" {
        w160 = T2 {"Mean"=99.0, " Std"=99.0, "Color Box"=16318226} ("Sensor")
        # "Initialize the front panel"
        n63 = stacked-sequence {
          tunnel: "Panel 1" -> [w168 w181]
          tunnel: w160 -> [w167 w180]
          tunnel: [w166 _] -> w159
          tunnel: "Panel 2" -> [_ _]
          tunnel: "Panel 3" -> [_ _]
          tunnel: [_ w178] -> w156
          frame #0 {
            n64 = for {
              tunnel: w168 -> [w171] mode=indexing
              tunnel: w167 -> [w170]
              tunnel: [w169] -> w166 mode=indexing
              n65 = for {
                tunnel: w171 -> [w177] mode=indexing
                tunnel: w170 -> [w176]
                tunnel: [w172] -> w169 mode=indexing
                n66 = Unbundle(w176) -> ("Mean"=w175:dbl, "Std"=w174:dbl, "Color Box"=w173:u32)
                n67 = Bundle By Name(cluster=w177, "Mean"=w175, "Std"=w174, "Color Box"=w173) -> (w172:T2)
              }
            }
          }
          frame #1 {
            n68 = for {
              N: 3 -> [_]
              tunnel: w181 -> [_] mode=indexing
              tunnel: w180 -> [w182]
              tunnel: [w182] -> w178 mode=indexing
            }
          }
        }
        "Temperatures" <- w156
        "Pressures" <- w156
        n69 = local write "Panel 1"(w159) -> ()
        n70 = local write "Panel 2"(w159) -> ()
        n71 = local write "Panel 3"(w159) -> ()
        n72 = call <vilib>:"Add State(s) to Queue__jki_lib_state_machine.vi"("State(s) in (\"\")"=w165) -> ("States Out"=w164:string)  [unwired: 14 in]
        "Power" <- w160
        "Tc Down" <- w160
      }
      frame "UI: Cursor Set" {
        # "Argument"
        n73 = case shown="\"Idle\", Default" w183 {
          tunnel: w185 -> [w190 w192]
          tunnel: [w189 w191] -> w184
          frame "Idle", Default {
            n74 = call <vilib>:"Unset Busy.vi"("error in (no error)"=w190) -> ("error out"=w189:errorcluster)  [unwired: 10 in]
          }
          frame "Busy" {
            n75 = call <vilib>:"Set Busy.vi"("error in (no error)"=w192) -> ("error out"=w191:errorcluster)  [unwired: 9 in, 1 out]
          }
        }
        n76 = call <vilib>:"Add State(s) to Queue__jki_lib_state_machine.vi"("State(s) in (\"\")"=w188) -> ("States Out"=w187:string)  [unwired: 14 in]
      }
      frame "UI: Front Panel State" {
        # "Set Front Panel Open or Closed\n(Usage: \"UI: Front Panel State >> Open|Close\")"
        n77 = Unbundle By Name(w195) -> ("Core.Current VI Reference"=w194:refnum<vi>)
        n78 = case shown="\"Open\", Default" w193 {
          tunnel: w197 -> [w203 w216]
          tunnel: [w205 w217] -> w196
          tunnel: w194 -> [w204 w214]
          frame "Open", Default {
            n79 = property class="VI"(reference=w204, error in=w203) -> (reference out=w201:refnum<vi>, error out=w202:errorcluster, "Front Panel.Open"=w200:bool)
            n80 = case shown="False" w200 {
              tunnel: [w208 w211] -> w205
              tunnel: w202 -> [w207 w211]
              tunnel: w201 -> [w206 _]
              frame False {
                n81 = invoke class="VI" method="FP.Open"(reference=w206, error in=w207, "Activate"=TRUE, "State"=T7."Maximized") -> (error out=w208:errorcluster)  [unwired: 1 in, 4 out]
              }
              frame True {
              }
            }
          }
          frame "Close" {
            n82 = property class="VI"(reference=w214, error in=w216) -> (reference out=w213:refnum<vi>, error out=w215:errorcluster, "Front Panel.Open"=w212:bool)
            n83 = case shown="True" w212 {
              tunnel: [w218 w221] -> w217
              tunnel: w215 -> [w218 w220]
              tunnel: w213 -> [_ w219]
              frame False {
              }
              frame True {
                n84 = invoke class="VI" method="FP.Close"(reference=w219, error in=w220) -> (error out=w221:errorcluster)  [unwired: 1 in, 2 out]
              }
            }
          }
        }
        n85 = call <vilib>:"Add State(s) to Queue__jki_lib_state_machine.vi"("State(s) in (\"\")"=w199) -> ("States Out"=w198:string)  [unwired: 14 in]
      }
      frame "---------- Macro ----------" {
        n86 = call <vilib>:"Add State(s) to Queue__jki_lib_state_machine.vi"("State(s) in (\"\")"=w225) -> ("States Out"=w224:string)  [unwired: 14 in]
      }
      frame "Macro: Initialize" {
        w226 = "Data: Initialize\nInitialize Core Data\nUI: Initialize\nUI: Front Panel State >> Open"  # Data: Initialize Initialize Core Data UI: Initialize UI: Front Panel State >> Open
        n87 = call <vilib>:"Add State(s) to Queue__jki_lib_state_machine.vi"("State(s) in Front (\"\")"=w226, "State(s) in (\"\")"=w230) -> ("States Out"=w229:string)  [unwired: 13 in]
      }
      frame "Macro: Exit" {
        n88 = Unbundle By Name(w237) -> ("Core.Close Panel on Exit?"=w236:bool)
        n89 = Select(t="UI: Front Panel State >> Close", s=w236, f="") -> (s? t:f=w233:string)
        n90 = call <vilib>:"Add State(s) to Queue__jki_lib_state_machine.vi"("State(s) in (\"\")"=w233, "State(s) at Back (\"\")"="Data: Cleanup\nExit") -> ("States Out"=w231:string)  [unwired: 13 in]
        n91 = call <vilib>:"Add State(s) to Queue__jki_lib_state_machine.vi"("State(s) in Front (\"\")"=w231, "State(s) in (\"\")"=w240) -> ("States Out"=w239:string)  [unwired: 13 in]
      }
      frame "---------- Main ----------" {
        n92 = call <vilib>:"Add State(s) to Queue__jki_lib_state_machine.vi"("State(s) in (\"\")"=w244) -> ("States Out"=w243:string)  [unwired: 14 in]
      }
      frame "Test: TCs" {
        n93 = call <vilib>:"Add State(s) to Queue__jki_lib_state_machine.vi"("State(s) in (\"\")"=w248) -> ("States Out"=w247:string)  [unwired: 14 in]
      }
      frame "------ TestDAQ ------" {
        n94 = call <vilib>:"Add State(s) to Queue__jki_lib_state_machine.vi"("State(s) in (\"\")"=w252) -> ("States Out"=w251:string)  [unwired: 14 in]
      }
      frame "TestDAQ: Gather" {
        n95 = Unbundle By Name(w259) -> ("Num Samples"=w253:i32, "Equipment Out"=w260)  [unwired: 1 out]
        n96 = for {
          N: w253 -> [_]
          tunnel: [w283] -> w256 mode=indexing
          shift-right: [w271] -> w261
          shift-left: w255 -> [w270]
          tunnel: w260 -> [w275]
          i -> [w282]
          n97 = local read "Calibration File Array"() -> (w269:dbl[][])
          n98 = control-ref of="Local Tank Display"() -> (w276:refnum<vi>)
          n99 = Multiply(x="Time Between Samples (Seconds)", y=u32 1000) -> (x*y=w272:u32)
          n100 = Wait (ms)(milliseconds to wait=w272) -> ()  [unwired: 1 out]
          n101 = call "HEWH Gather Test Data.vi"("Equipment"=w275, "Tank Display Ref"=w276, "Calibration Coefficients"=w269, "error in (no error)"=w270) -> ("Output Data"=w278:string[][], "error out"=w271:errorcluster)  [unwired: 7 in, 3 out]
          "Output Data" <- w278
          n102 = Array Size(array=w278) -> (size(s)=w281:i32[])
          n103 = Array Max & Min(array=w281) -> (max value=w280:i32)  [unwired: 3 out]
          n104 = Index Array(array=w278, index (row)=1 ("index")) -> (element=w277:string[])  [unwired: 1 in]
          n105 = Reshape Array(w277, w280) -> (w284:string[])
          n106 = Fract/Exp String To Number(string=w284) -> (number=w283:dbl[])  [unwired: 3 in, 1 out]
          "Data Sample" <- w282
        }
        n107 = call <vilib>:"Add State(s) to Queue__jki_lib_state_machine.vi"("State(s) in (\"\")"=w263) -> ("States Out"=w262:string)  [unwired: 14 in]
        n108 = Transpose 2D Array(2D array=w256) -> (transposed array=w254:dbl[][])
        "Raw Data" <- w254
        n109 = for {
          tunnel: [w266] -> w258 mode=indexing
          tunnel: w254 -> [w264] mode=indexing
          n110 = call <vilib>:"Std Deviation and Variance.vi"("X"=w264) -> ("mean"=w268:dbl, "standard deviation"=w267:dbl)  [unwired: 1 in, 1 out]
          n111 = Bundle By Name(cluster=T2 {"Mean"=0.0, " Std"=0.0, "Color Box"=5373696} ("Sensor"), "Mean"=w268, "Std"=w267) -> (w266:T2)
        }
        n112 = Bundle By Name(cluster=w259, "Test Data Array"=w258) -> (w257:T8)
      }
      frame "TestDAQ: Sort" {
        n113 = Unbundle By Name(w286) -> ("Test Data Array"=w285:T2[])
        n114 = stacked-sequence {
          tunnel: w285 -> [w298 w320 w341 w361]
          frame #0 {
            n115 = local read "Panel 1"() -> (w290:T2[][])
            n116 = Array Subset(array=w298, index=23, length=6) -> (w294:T2[])
            n117 = Array Subset(array=w298, index=22, length=1) -> (w297:T2[])
            n118 = Array Subset(array=w298, index=30, length=3) -> (w296:T2[])
            n119 = Array Subset(array=w298, index=39, length=2) -> (w295:T2[])
            n120 = Build Array (concatenate)(w297, w296, w295) -> (w293:T2[])
            n121 = Replace Array Subset(array=w290, new element=w294, index (row)=0) -> (w311:T2[][])  [unwired: 1 in]
            n122 = Replace Array Subset(array=w311, new element=w293, index (row)=1) -> (w309:T2[][])  [unwired: 1 in]
            n123 = Array Subset(array=w298, index=41, length=6) -> (w292:T2[])
            n124 = Replace Array Subset(array=w309, new element=w292, index (row)=2) -> (w291:T2[][])  [unwired: 1 in]
            n125 = local write "Panel 1"(w291) -> ()
          }
          frame #1 {
            n126 = Array Subset(array=w320, index=48, length=6) -> (w323:T2[])
            n127 = local read "Panel 2"() -> (w314:T2[][])
            n128 = Replace Array Subset(array=w314, new element=w323, index (row)=0) -> (w328:T2[][])  [unwired: 1 in]
            n129 = Array Subset(array=w320, index=54, length=6) -> (w319:T2[])
            n130 = Replace Array Subset(array=w328, new element=w319, index (row)=1) -> (w326:T2[][])  [unwired: 1 in]
            n131 = Array Subset(array=w320, index=60, length=6) -> (w318:T2[])
            n132 = Replace Array Subset(array=w326, new element=w318, index (row)=2) -> (w317:T2[][])  [unwired: 1 in]
            n133 = local write "Panel 2"(w317) -> ()
          }
          frame #2 {
            (unwired) 6 ("length")
            n134 = Array Subset(array=w341, index=71, length=6) -> (w336:T2[])
            n135 = local read "Panel 3"() -> (w331:T2[][])
            n136 = Replace Array Subset(array=w331, new element=w336, index (row)=0) -> (w332:T2[][])  [unwired: 1 in]
            n137 = Array Subset(array=w341, index=77) -> (w335:T2[])  [unwired: 1 in]
            n138 = Array Subset(array=w341, index=47, length=1) -> (w338:T2[])
            n139 = Array Subset(array=w341, index=66, length=5) -> (w337:T2[])
            n140 = Replace Array Subset(array=w332, new element=w335, index (row)=1) -> (w347:T2[][])  [unwired: 1 in]
            n141 = Build Array (concatenate)(w338, w337) -> (w334:T2[])
            n142 = Replace Array Subset(array=w347, new element=w334, index (row)=2) -> (w333:T2[][])  [unwired: 1 in]
            n143 = local write "Panel 3"(w333) -> ()
          }
          frame #3 {
            # "Temperatures"
            # "Pressures"
            n144 = Index Array(array=w361, index=15) -> (element=w359:T2)
            n145 = Array Subset(array=w361, index=17, length=3) -> (w358:T2[])
            n146 = Index Array(array=w361, index=29) -> (element=w360:T2)
            n147 = Index Array(array=w361, index #1=35 ("index"), index #2=33 ("index"), index #3=34 ("length")) -> (element #1=w354:T2, element #2=w353:T2, element #3=w352:T2)
            n148 = local write "Power"(w359) -> ()
            n149 = local write "Pressures"(w358) -> ()
            n150 = local write "Tc Down"(w360) -> ()
            n151 = Build Array(w354, w353, w352) -> (w351:T2[])
            n152 = local write "Temperatures"(w351) -> ()
          }
        }
        n153 = call <vilib>:"Add State(s) to Queue__jki_lib_state_machine.vi"("State(s) in (\"\")"=w289) -> ("States Out"=w288:string)  [unwired: 14 in]
      }
      frame "TestDAQ: Verify" {
        # "This routine checks to see if the average values (avg and stdev) is within specification"
        n154 = local read "Temperatures"() -> (w366:T2[])
        n155 = local read "Pressures"() -> (w367:T2[])
        n156 = local read "Panel 1"() -> (w370:T2[][])
        n157 = local read "Panel 2"() -> (w369:T2[][])
        n158 = local read "Panel 3"() -> (w368:T2[][])
        n159 = stacked-sequence {
          tunnel: w369 -> [_ w383 _ _ _]
          tunnel: w370 -> [w375 _ _ _ _]
          tunnel: w368 -> [_ _ w389 _ _]
          tunnel: w367 -> [_ _ _ w400 _]
          tunnel: w366 -> [_ _ _ _ w405]
          frame #0 {
            n160 = for {
              tunnel: [w381] -> w376 mode=indexing
              tunnel: w375 -> [w380] mode=indexing
              n161 = call "HEWH Color Check.vi"("Min OK Val"="TC Min OK Val", "Max OK Val"="TC Max OK Val", "StDev Thresh"="StDev Thresh", "Panel 1"=w380) -> ("Array"=w381:T2[])  [unwired: 7 in]
            }
            n162 = local write "Panel 1"(w376) -> ()
          }
          frame #1 {
            n163 = for {
              tunnel: w383 -> [w388] mode=indexing
              tunnel: [w384] -> w382 mode=indexing
              n164 = local read "TC Max OK Val"() -> (w386:dbl)
              n165 = local read "TC Min OK Val"() -> (w385:dbl)
              n166 = local read "StDev Thresh"() -> (w387:dbl)
              n167 = call "HEWH Color Check.vi"("Min OK Val"=w385, "Max OK Val"=w386, "StDev Thresh"=w387, "Panel 1"=w388) -> ("Array"=w384:T2[])  [unwired: 7 in]
            }
            n168 = local write "Panel 2"(w382) -> ()
          }
          frame #2 {
            n169 = for {
              tunnel: w389 -> [w395] mode=indexing
              tunnel: [w394] -> w390 mode=indexing
              n170 = local read "TC Max OK Val"() -> (w392:dbl)
              n171 = local read "TC Min OK Val"() -> (w391:dbl)
              n172 = local read "StDev Thresh"() -> (w393:dbl)
              n173 = call "HEWH Color Check.vi"("Min OK Val"=w391, "Max OK Val"=w392, "StDev Thresh"=w393, "Panel 1"=w395) -> ("Array"=w394:T2[])  [unwired: 7 in]
            }
            n174 = local write "Panel 3"(w390) -> ()
          }
          frame #3 {
            n175 = local read "StDev Thresh"() -> (w399:dbl)
            n176 = call "HEWH Color Check.vi"("Min OK Val"="PSI Min OK", "Max OK Val"="PSI Max OK", "StDev Thresh"=w399, "Panel 1"=w400) -> ("Array"=w396:T2[])  [unwired: 7 in]
            n177 = local write "Pressures"(w396) -> ()
          }
          frame #4 {
            n178 = local read "StDev Thresh"() -> (w403:dbl)
            n179 = call "HEWH Color Check.vi"("Min OK Val"="RTD Min OK", "Max OK Val"="RTD Max OK", "StDev Thresh"=w403, "Panel 1"=w405) -> ("Array"=w404:T2[])  [unwired: 7 in]
            n180 = local write "Temperatures"(w404) -> ()
          }
        }
        n181 = call <vilib>:"Add State(s) to Queue__jki_lib_state_machine.vi"("State(s) in (\"\")"=w374) -> ("States Out"=w373:string)  [unwired: 14 in]
      }
      frame "Calibration" {
        n182 = local read "Select Panel to Calibrate"() -> (w408:enum16{"Panel 1", "Panel 2", "Panel 3"})
        n183 = case shown="\"Panel 1\", Default" w408 {
          tunnel: [w413 w414 w415] -> w409
          frame "Panel 1", Default {
            n184 = local read "Panel 1"() -> (w413:T2[][])
          }
          frame "Panel 2" {
            n185 = local read "Panel 2"() -> (w414:T2[][])
          }
          frame "Panel 3" {
            n186 = local read "Panel 3"() -> (w415:T2[][])
          }
        }
        n187 = stacked-sequence {
          tunnel: w409 -> [_ w454]
          tunnel: w407 -> [w416 _]
          tunnel: [w416 _] -> w406
          frame #0 {
            n188 = local read "Degrees F"() -> (w417:dbl)
            n189 = local write "Temperature"(w417) -> ()
          }
          frame #1 {
            w451 = 0 ("disabled index (col)")
            n190 = for {
              tunnel: w454 -> [w460] mode=indexing
              tunnel: [w459] -> w450 mode=indexing
              n191 = for {
                tunnel: w460 -> [w464] mode=indexing
                tunnel: [w462] -> w459 mode=indexing
                n192 = Unbundle By Name(w464) -> ("Mean"=w463:dbl)
                n193 = local read "Temperature"() -> (w461:dbl)
                n194 = Subtract(x=w461, y=w463) -> (x-y=w462:dbl)
              }
            }
            n195 = local read "Tc Down"() -> (w426:T2)
            n196 = local read "Temperature"() -> (w424:dbl)
            n197 = local read "Temperature"() -> (w428:dbl)
            n198 = Unbundle By Name(w426) -> ("Mean"=w425:dbl)
            n199 = Subtract(x=w424, y=w425) -> (x-y=w423:dbl)
            n200 = Number To Fractional String(number=w428, precision (6)=i16 0) -> (F-format string=w436:string)  [unwired: 2 in]
            n201 = Number To Fractional String(number=w423) -> (F-format string=w422:string)  [unwired: 3 in]
            n202 = Delete From Array(array=w450, index (row)=w451) -> (deleted portion=w449:dbl[], array with subset deleted=w453:dbl[][])  [unwired: 2 in]
            n203 = Concatenate Strings("TC Setpoint " ("string"), w436, "  Deg F" ("string"), "," ("string")) -> (w431:string)
            n204 = Delete From Array(array=w453, index (row)=w451) -> (deleted portion=w448:dbl[], array with subset deleted=w452:dbl[][])  [unwired: 2 in]
            n205 = Delete From Array(array=w452, index (row)=w451) -> (deleted portion=w447:dbl[])  [unwired: 2 in, 1 out]
            n206 = Build Array (concatenate)(w449, w448, w447) -> (w441:dbl[])
            n207 = Array Size(array=w441) -> (size(s)=w440:i32)
            n208 = Build Array(w441) -> (w445:dbl[][])
            n209 = local read "Calibration File Path"() -> (w418:path)
            n210 = Transpose 2D Array(2D array=w445) -> (transposed array=w446:dbl[][])
            n211 = Array To Spreadsheet String(delimiter (Tab)="," ("delimiter (\\t)"), array=w446, 3:"%.3f" ("format string")) -> (spreadsheet string=w442:string)
            n212 = for {
              N: w440 -> [_]
              shift-right: [w455] -> w432
              shift-left: w442 -> [w456]
              n213 = Search and Replace String(input string=w456, search string="\r\n", replace string="," ("replace string (\"\")")) -> (result string=w455:string)  [unwired: 5 in, 3 out]
            }
            n214 = Concatenate Strings(w431, w432, w422, "," ("string"), "\\n" ("string"), "\r\n") -> (w430:string)
            n215 = Build Array(w430) -> (w429:string[])
            n216 = call-poly <vilib>:"Write To Spreadsheet File.vi"("delimiter (\\t)"="," ("delimiter (\\t)"), "format (%s)"="%s", "append to file? (new file:F)"=TRUE, "1D data"=w429, "file path (dialog if empty)"=w418) -> ()  [unwired: 3 in, 1 out]
          }
        }
        n217 = call <vilib>:"Add State(s) to Queue__jki_lib_state_machine.vi"("State(s) in (\"\")"=w412) -> ("States Out"=w411:string)  [unwired: 14 in]
      }
    }
  }
